vi "Main_MaintenanceCounters.vi"() -> ()   [LabVIEW 2017]
panel:
  in  "LastCycleTimeCluster":cluster{"MachineName":string, "LastHour":string}
  out "LastCycleTimePath":path
  in  "CycleTimeArray":T1(array[cluster])
  in  "LastSeconds":i32
  out "ThisAppPath":path
  out "ModificationArray":string[](array[string])
  out "HourResetEnabled":string
  out "CycleCountHour":T2
  in  "ArrayCycleCountHour":T3(array[cluster])
  out "UserLevel":i32
  out "ServerConnectionStatus":string
  out "Line Name":string
  out "Array_BooleanMemoryPLC":T4(array[cluster])
  out "UserLogged":string
  in  "FormatCountersConfigArray":T5(array[cluster]) {"StoppageAlarmCounter" format="%#_6f"; "PreparationAlarmCounter" format="%#_6f"}
  out "CycleTimeCluster":T6
  out "Table Control":string[][](table)
  out "ConnectionCluster":cluster{"Connection":bool, "MachineName":string}
  out "UDT_1":T7
  in  "CountersConfiguration":T8
  out "CountersConfigMerged":T5(array[cluster])
  out "CounterLineName Path":path
  in  "Tab":T9(tab)
  in  "RefreshLists":bool
  in  "Selector_P#-Description":u16(ring) items=["104567 - Spinning Belt", "108724 - Emergency Stop", "105855 - Helicoil", "101415 - Inductive Sensor", "101111 - Magnetic Sensor"]
  in  "Selector_MachineSpareParts":u16(ring) items=["MA530", "MA520", "MA500-3", "MA500-2", "MA500-1", "MA490-2", "MA490-1", "MA475", "MA470", "MA455", "MA336", "MA335", "SNX2030"]
  out "PathLocationMachineImage":path
  out "PathSparePartImage":path
  out "Image_LocationInMachine":T10(plugin-control)
  out "Image_SparePart":T10(plugin-control)
  in  "ModelName":u16(ring) items=["F042", "F070", "F0AU"]
  in  "Add Button":bool
  out "Description":string
  out "Tool Crib PN":string
  in  "SearchSpareParts":bool
  in  "CountersConfigArray":T5(array[cluster]) {"StoppageAlarmCounter" format="%#_6f"; "PreparationAlarmCounter" format="%#_6f"}
  in  "RefreshCountersConfig":bool
  in  "SaveCountersConfig":bool
  out "Counters Configuration Path":path
  in  "MachineNameID":u16(ring) items=["MA530", "MA520", "MA500-3", "MA500-2", "MA500-1", "MA490-2", "MA490-1", "MA475", "MA470", "MA455", "MA336", "MA335", "SNX2030"]
  in  "PLC Connection Array":T11(array[cluster]) {"PLC Type" items=["Keyence", "Allen Bradley", "Mitsubishi", "Panasonic", "Siemens"]}
  out "PLC Configuration Path":path
  in  "SavePLCConfig":bool
  in  "RefreshPLCConfig":bool
  in  "CreateTables":bool
  in  "EditUser":bool
  in  "GeneralParametersArray":cluster{"Parameter":string, "Value":string}[](array[cluster])
  in  "LoadDefaultConfig":bool
  in  "RemoveUser":bool
  in  "Logout":bool
  in  "Login":bool
  in  "AddUser":bool
  in  "GDrive":bool
  out "GeneralConfigPath":path
  in  "RefreshGeneralConfig":bool
  in  "SaveGeneralConfig":bool
  in  "ShowParetto":bool
  out "CycleTimeMonitor":T12(array[cluster])
  out "CycleTimePath":path
  out "legend":string[][](table)
  in  "Tab Control":T13(tab)
  in  "DictionaryArray":T14(array[cluster]) {"LifeCycle" format="%#_6f"}
  out "PathDictionary":path
  in  "SaveDictionary":bool
  in  "RefreshDictionary":bool
  in  "ResetAlarmButton":bool
  in  "QualityLogin":bool
  in  "MaintenanceLogin":bool
  in  "ResetAlarm":bool[](array[boolean])
  out "ArrayAlarm":bool[](array[boolean])
  out "OnlineStations":T15(array[cluster])
  in  "Counters Monitor Array":T16(array[cluster])
  out "CurrentCountersPath":path
  in  "Count Signal":bool[](array[boolean])
  in  "SaveCurrentCounter":bool
  in  "RefreshCurrentCounter":bool
  in  "Sort":bool
  out "Hour":string
  in  "stop":bool
  # "Cycles Based Maintenance"
  # "User"
  # "Line"
  # "Nidec Server Connection"
  # "Refresh Lists"
  # "Select Machine"
  # "Select PartNumber - Description"
  # "Location in the Machine"
  # "Spare Part Image"
  # "These paths are calculated automatically"
  # "Machine Name"
  # "Tool Crib P#"
  # "Description"
  # "SP1"
  # "SP2"
  # "Search Result"
  # "Model"
  # "Note:\nSP1 = Is the setpoint for the counter when the \nmachine will alert to prepare the replacement of\nthe component. This gives the technician time\nto get parts together.\n\nSP2 = Is the setpoint for the counter when the\nmachine will stop the operation until the part is \nreplaced, the operation can only be reset until\na quality employee comes to unlock with its \nuser and password."
  # "USER LEVEL 3 OR ABOVE TO ENABLE THIS CONFIGURATION IS NEEDED."
  # "Add the option to connect by serial port"
  # "Count Signal"
  # "Alarm Signal"
  # "Alarm Message"
  # "Machine Name"
  # "PLC Address"
  # "PLC Type"
  # "Value"
  # "Parameter"
  # "User Level 5 Requiered to View General Parameters"
  # "User Management"
  # "Idle Time: Is the maximum waiting time before a breakdown incidence is\nconsidered and created."
  # "Escalation Time: Is the maximum waiting time before sending an email \nto the escalation chain."
  # "Cycle Time Monitor"
  # "Cycle Time Monitor"
  # "Note: \nTo add a machine in this list of counters configuration it must be firt added in the PLC Connection tab."
  # "The SubAssembly can be either EOL, Motor, Stator, Rotor Etc, This is used to be able to crate several tables for the same line."
  # "buscar multiplos de ciclos para que coincidan \n\nestudiar investigacion de operaciones\n\nAgrupar las maquinas que trabajan en conjunto para agrupar tareas de mantenimiento.\nCambiar el metodo de seleccion de memorias de PLC usando solo strings para hacerlos universales."
  # "Nota para desarrollador: Revisar que al cerrar la incidencia se apague la alarma y se resetee el contador"
  # "1. Save counters to be loaded in the last state when the app starts up.\n\n2.Algorithm to read PLC counter values.\nthe key will be to set the signal from the PLC and reset from LabVIEW and the machine won't be able to start the new signal if the application has not been reset the previous one.\n\n3. Autosort getting the red status all the way up.\n\n4. Check cyle time between parts (The count signal must is the same for all the components in the same machine)"
  # "Component"
  # "Cycle Life"
  # "Manual"
  # "Un calculador de tiempo de vida en ciclos, que dependa del tipo de componente para calcular de acuerdo a la aplicacion.\n\npor ejemplo un slider, su tiempo de vida en es km de recorrido, midiendo cuanto se desplaza en cada movimiento, y cuantos desplazamientos hace por ciclo, se puede predecir, a los cuantos\nciclos va a fallar."
  # "Version:\nCBM V1.1\n03/03/2022 - 11:00\nEdgar Cruz\nMaintenance"
  # "Release Notes:\nV1.1 Will be able to support different PLC. since previous version only supports Keyence.\nFirts instance will be Allen Bradly to handle MK100."
  # "MachineName"
  # "Tool Crib"
  # "ComponentName"
  # "Counter SetPoint"
  # "Actual"
  # "Status"
  # "Online Stations"
  # "Current Hour"
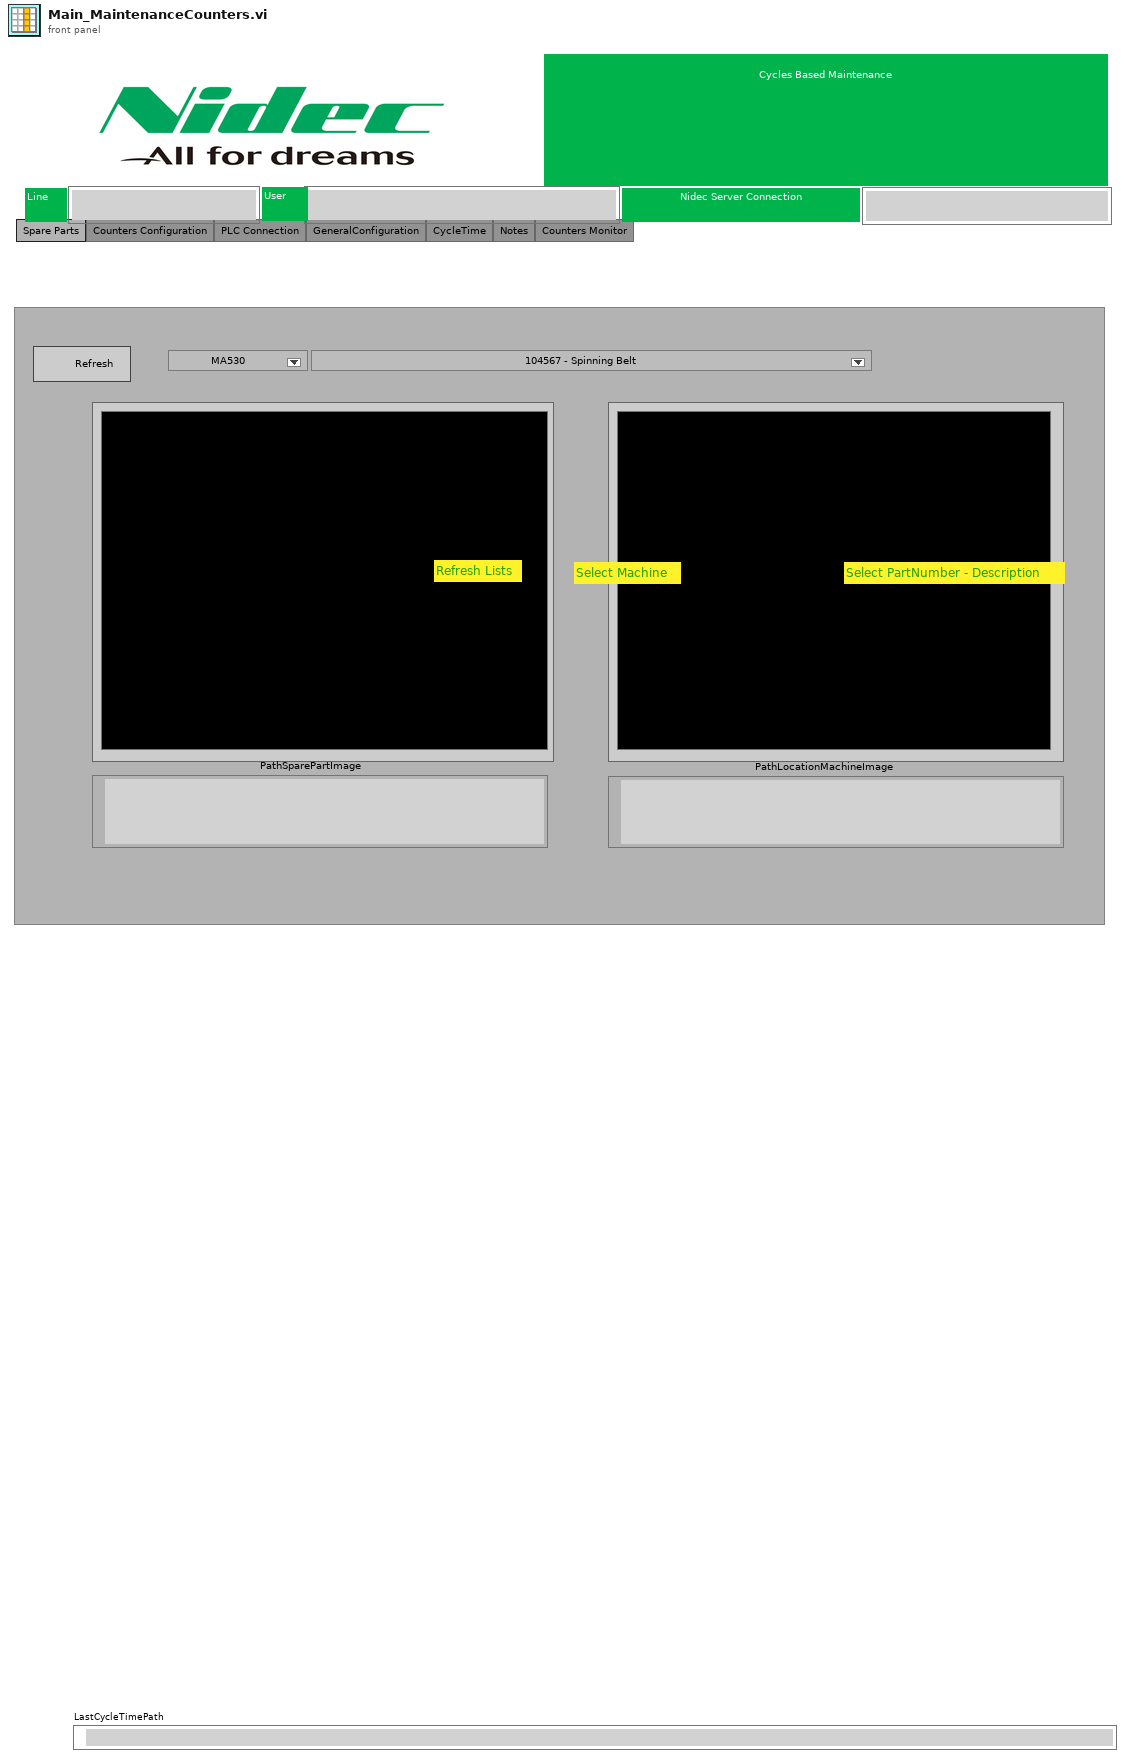
[diagram p1: front panel]
types:
  T1 = cluster{"MachineName":string, "LastHour":string}[]
  T2 = cluster{"MachineName":string, "HourLastCycle":string}
  T3 = cluster{"MachineName":string, "HourLastCycle":string}[]
  T4 = cluster{"PLC_Signal":bool, "MachineName":string}[]
  T5 = cluster{"ToolCribPartNumber":string, "ComponentName":string, "PreparationAlarmCounter":dbl, "StoppageAlarmCounter":dbl}[]
  T6 = cluster{"Connection":bool, "MachineName":string, "CycleTime":dbl}
  T7 = cluster{"ToolCribPartNumber":string, "ComponentName":string, "PreparationAlarmCounter":dbl, "StoppageAlarmCounter":dbl, "MachineName":string}
  T8 = cluster{"MachineName":string, "ComponentName":string, "StoppageAlarmCounter":dbl, "CurrentCount":dbl, "StatusColorBox":u32, "ToolCribPartNumber":string}
  T9 = enum32{"Spare Parts", "Counters Configuration", "PLC Connection", "GeneralConfiguration", "CycleTime", "Notes", "Counters Monitor"}
  T10 = typedef "IMAQ Image.ctl" = refnum<image>
  T11 = cluster{"MachineName":string, "PLC Address":string, "PLC Type":u16, "MemoryNumber1":string, "MemoryNumber2":string, "MemoryNumber3":string}[]
  T12 = cluster{"Connection":bool, "MachineName":string, "CycleTime":dbl}[]
  T13 = enum32{"Notes", "Dictionary", "Calculator", "Version Information"}
  T14 = cluster{"ComponentDescription":string, "LifeCycle":dbl, "ManualPDF":string}[]
  T15 = cluster{"Connection":bool, "MachineName":string}[]
  T16 = cluster{"MachineName":string, "ComponentName":string, "StoppageAlarmCounter":i32, "CurrentCount":i32, "StatusColorBox":u32, "ToolCribPartNumber":string}[]
  T17 = cluster{"ToolCribPartNumber":string, "ComponentName":string, "PreparationAlarmCounter":dbl, "StoppageAlarmCounter":dbl, "MachineName":string}[]
  T18 = cluster{"MachineName":string, "ComponentName":string, "StoppageAlarmCounter":i32, "CurrentCount":i32, "StatusColorBox":u32, "ToolCribPartNumber":string}
  T19 = enum8{"Enabled", "Disabled", "Disabled and Grayed Out"}
  T20 = typedef "Image Type" = u32
  T21 = cluster{"ToolCribPartNumber":string, "ComponentName":string, "PreparationAlarmCounter":dbl, "StoppageAlarmCounter":dbl}
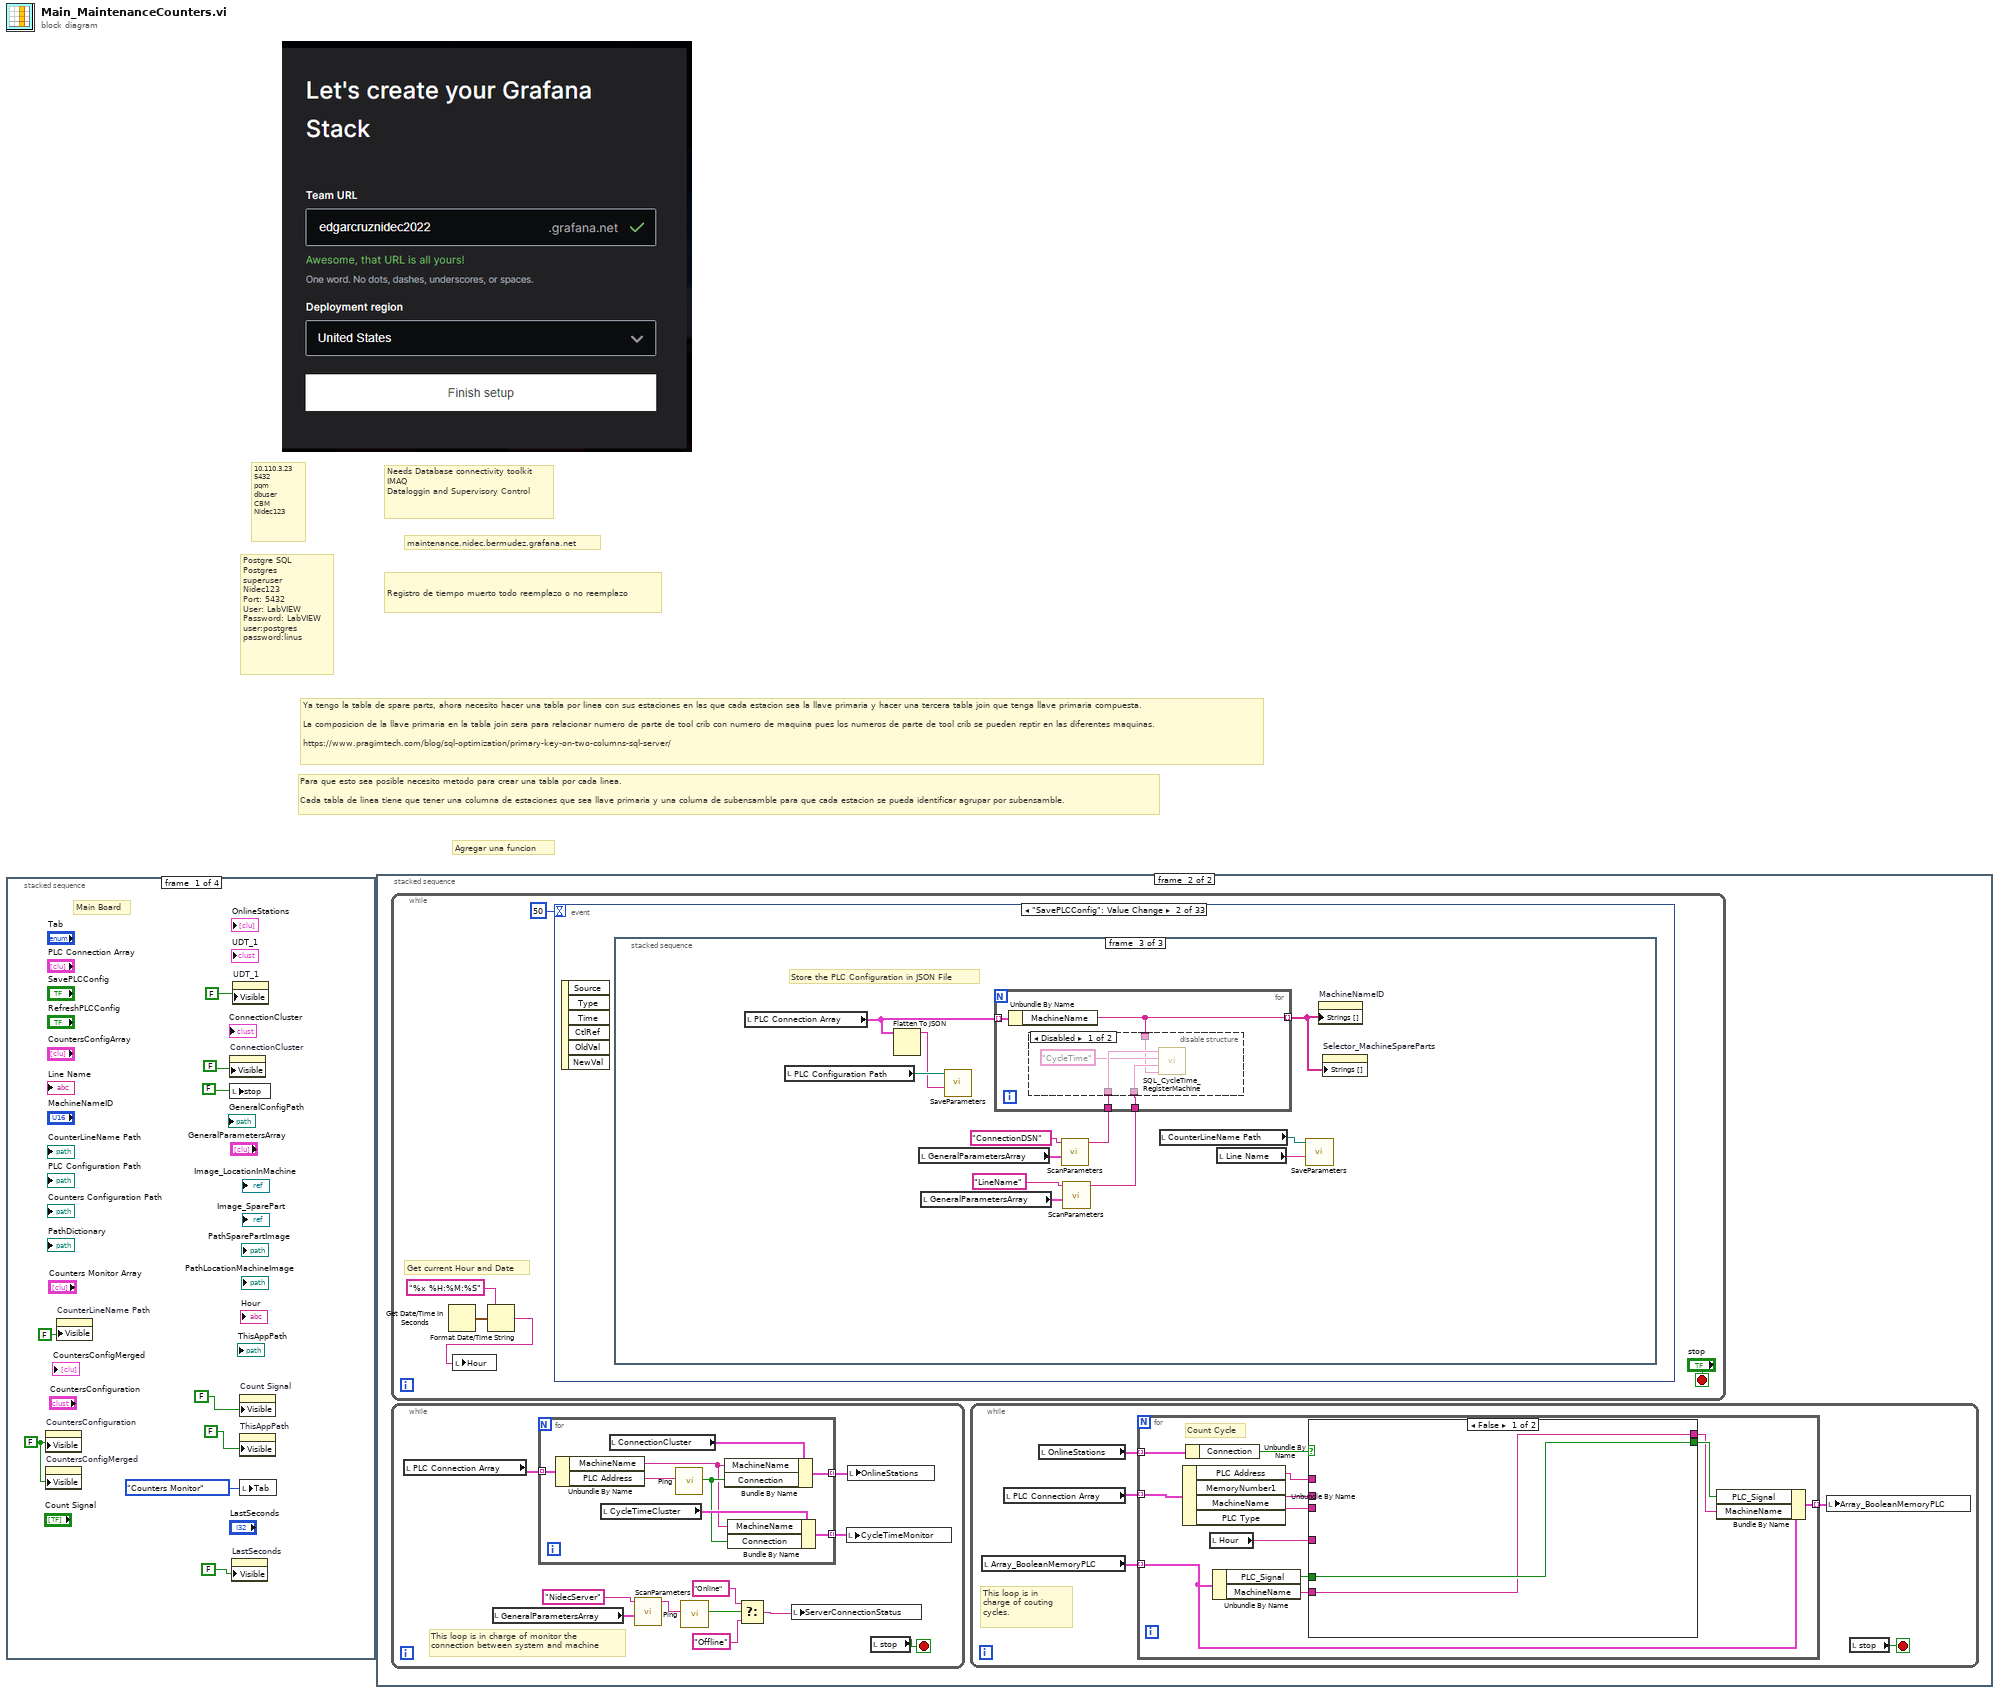
[diagram p0: block diagram]
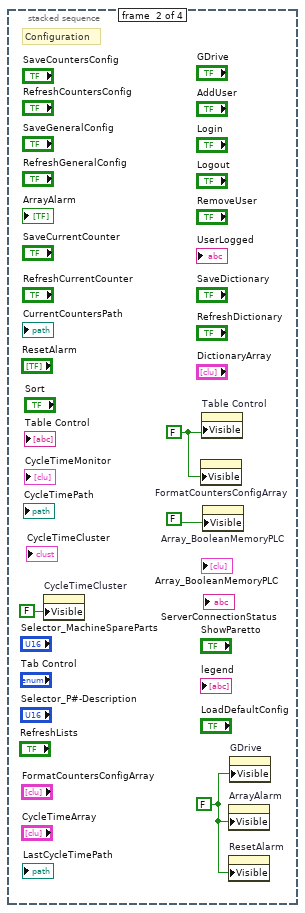
[diagram p2: hidden frame]
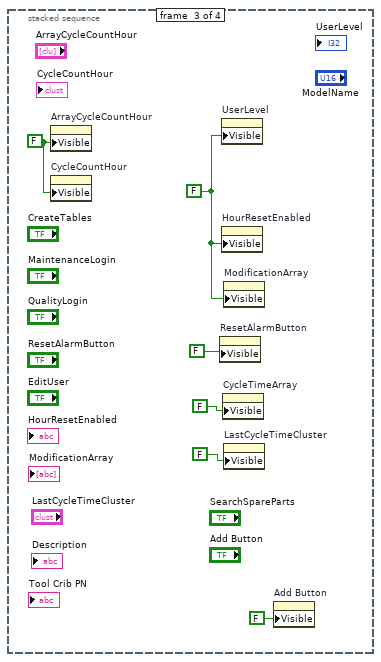
[diagram p3: hidden frame]
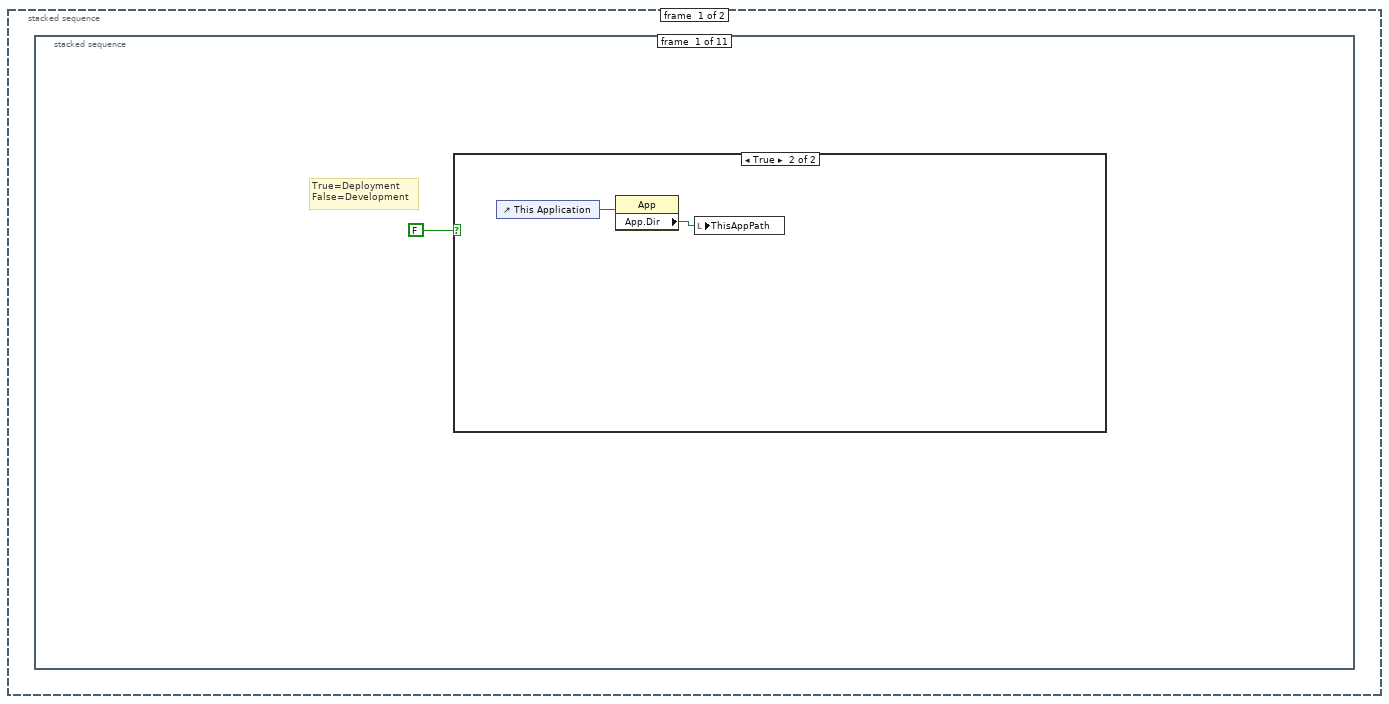
[diagram p5: hidden frame]
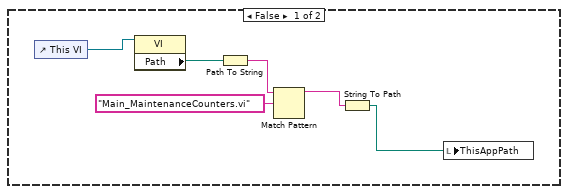
[diagram p6: hidden frame]
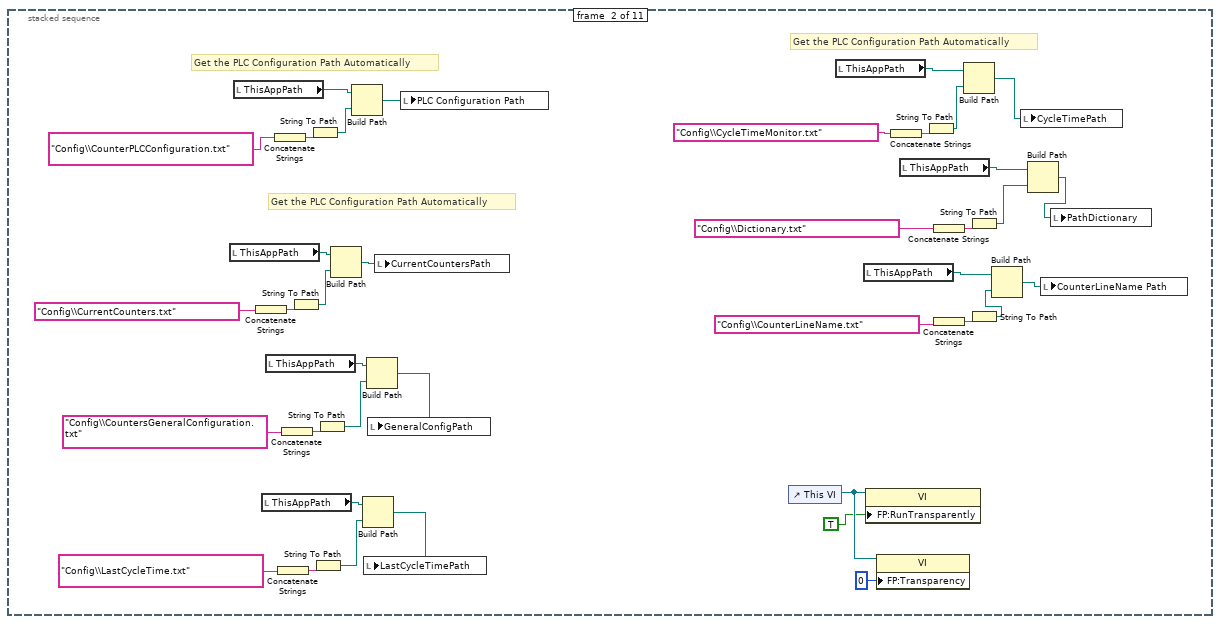
[diagram p7: hidden frame]
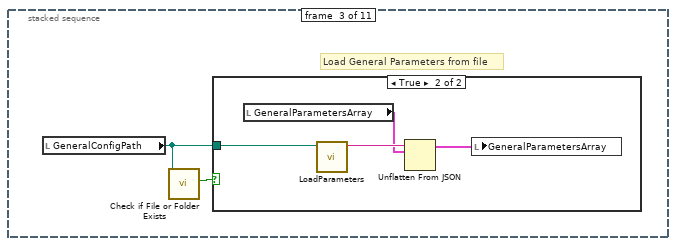
[diagram p8: hidden frame]
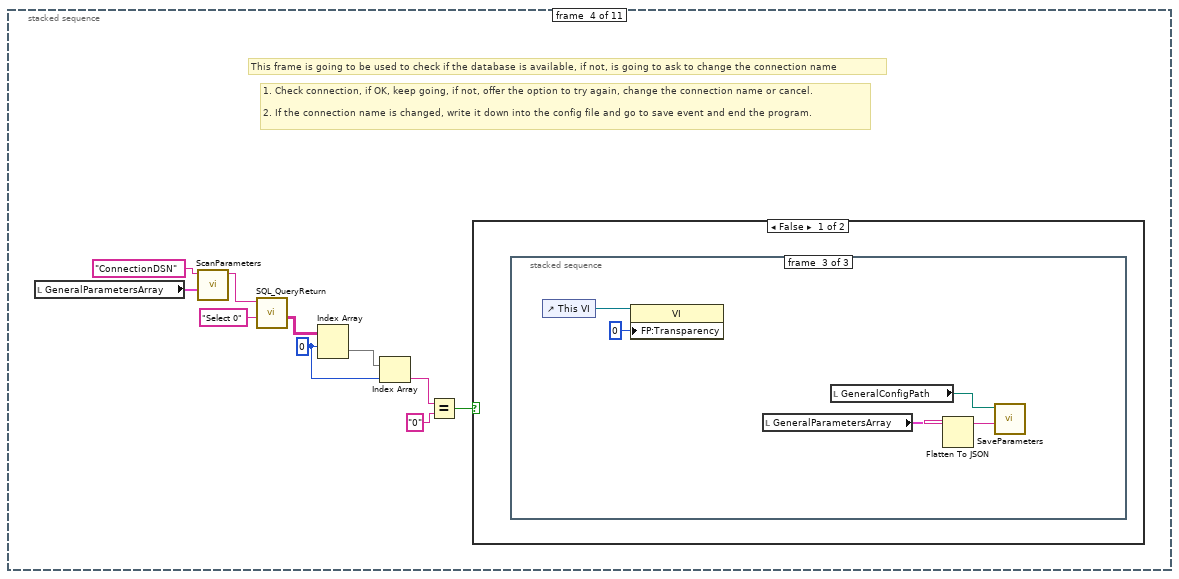
[diagram p10: hidden frame]
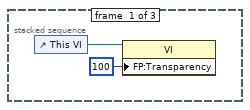
[diagram p11: hidden frame]
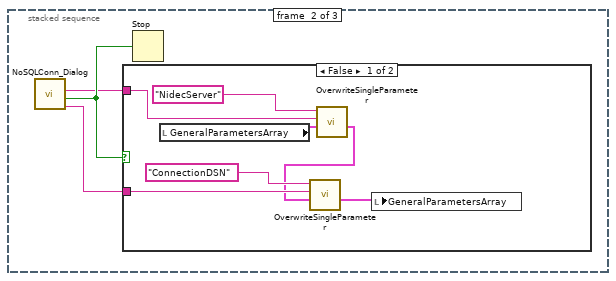
[diagram p12: hidden frame]
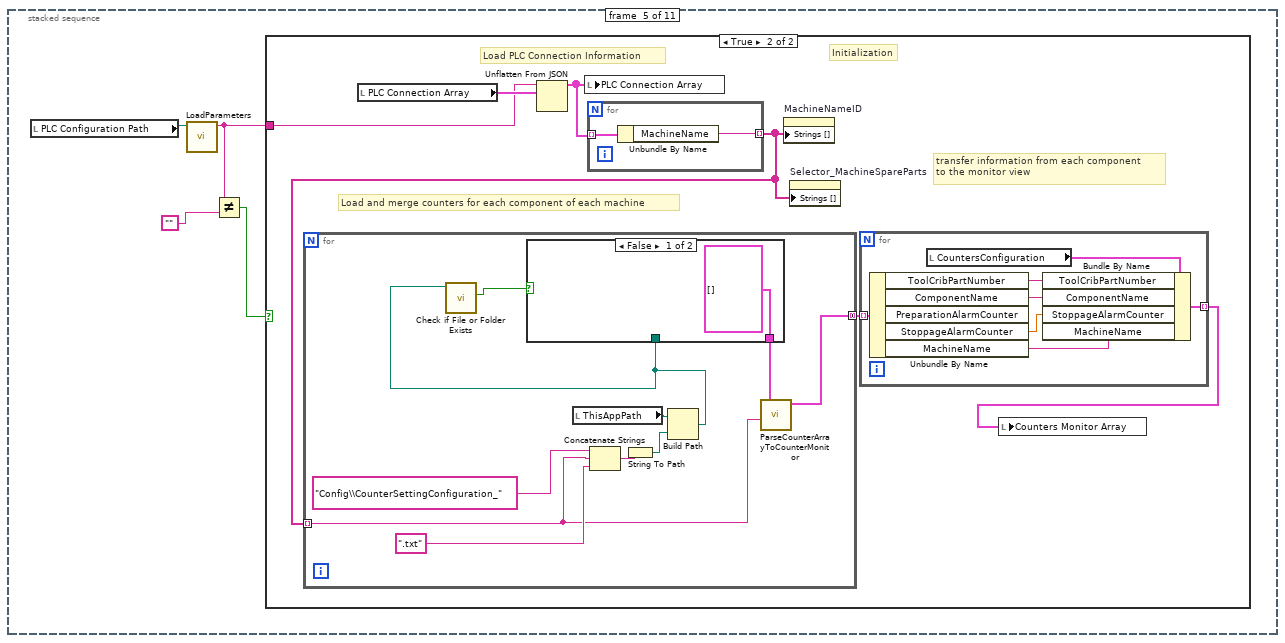
[diagram p15: hidden frame]
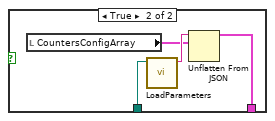
[diagram p17: hidden frame]
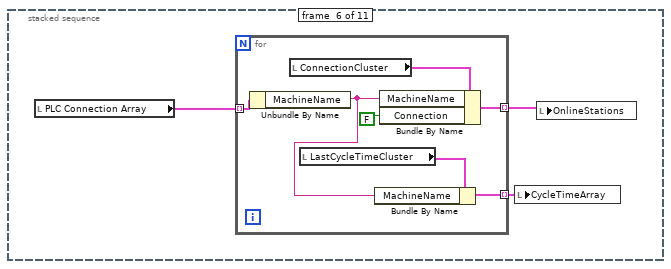
[diagram p18: hidden frame]
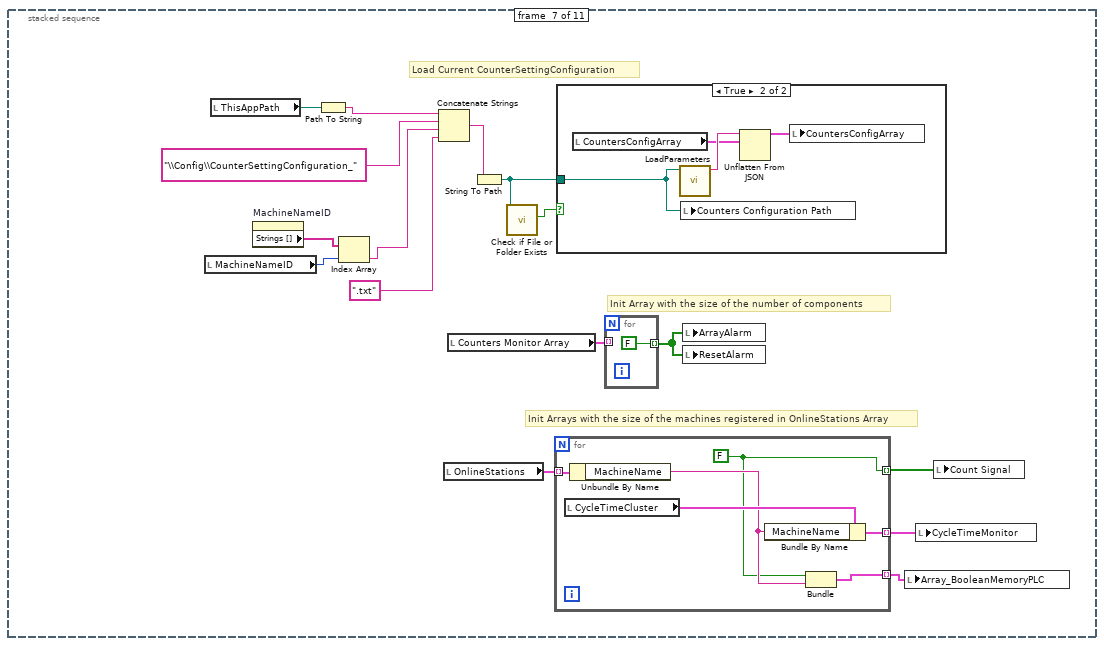
[diagram p19: hidden frame]
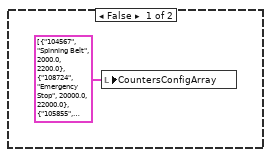
[diagram p20: hidden frame]
diagram:
  # "Agregar una funcion"
  # "Para que esto sea posible necesito metodo para crear una tabla por cada linea.\n\nCada tabla de linea tiene que tener una columna de estaciones que sea llave primaria y una columa de subensamble para que cada estacion se pueda identificar agrupar por subensamble."
  # "Ya tengo la tabla de spare parts, ahora necesito hacer una tabla por linea con sus estaciones en las que cada estacion sea la llave primaria y hacer una tercera tabla join que tenga llave primaria compuesta.\n\nLa composicion de la llave primaria en la tabla join sera para relacionar numero de parte de tool crib con numero de maquina pues los numeros de parte de tool crib se pueden reptir en las diferentes maquinas.\n\nhttps://www.pragimtech.com/blog/sql-optimization/primary-key-on-two-columns-sql-server/"
  # "10.110.3.23\n5432\npqm\ndbuser\nCBM\nNidec123"
  # "maintenance.nidec.bermudez.grafana.net"
  # "Needs Database connectivity toolkit\nIMAQ\nDataloggin and Supervisory Control"
  # "Registro de tiempo muerto todo reemplazo o no reemplazo"
  # "Postgre SQL \nPostgres\nsuperuser\nNidec123\nPort: 5432\nUser: LabVIEW\nPassword: LabVIEW\nuser:postgres\npassword:linus"
  n1 = stacked-sequence {
    frame #0 {
      w8 = FALSE
      # "Main Board"
      n2 = property on="CountersConfiguration" class="Clust (strict)"("Visible"=w8) -> ()  [unwired: 2 in, 2 out]
      n3 = property on="CountersConfigMerged" class="Arr (strict)"("Visible"=w8) -> ()  [unwired: 2 in, 2 out]
      n4 = property on="CounterLineName Path" class="Path"("Visible"=FALSE) -> ()  [unwired: 2 in, 2 out]
      n5 = property on="ConnectionCluster" class="Clust (strict)"("Visible"=FALSE) -> ()  [unwired: 2 in, 2 out]
      n6 = local write "stop"(FALSE ("stop")) -> ()
      n7 = property on="LastSeconds" class="DigNum (strict)"("Visible"=FALSE) -> ()  [unwired: 2 in, 2 out]
      n8 = property on="UDT_1" class="Clust (strict)"("Visible"=FALSE) -> ()  [unwired: 2 in, 2 out]
      n9 = property on="Count Signal" class="Arr (strict)"("Visible"=FALSE) -> ()  [unwired: 2 in, 2 out]
      n10 = property on="ThisAppPath" class="Path"("Visible"=FALSE) -> ()  [unwired: 2 in, 2 out]
      n11 = local write "Tab"(T9."Counters Monitor" ("Tab")) -> ()
    }
    frame #1 {
      w11 = FALSE ("Visible")
      w12 = FALSE ("Visible")
      # "Configuration"
      n12 = property on="CycleTimeCluster" class="Clust (strict)"("Visible"=FALSE) -> ()  [unwired: 2 in, 2 out]
      n13 = property on="FormatCountersConfigArray" class="Arr (strict)"("Visible"=w12) -> ()  [unwired: 2 in, 2 out]
      n14 = property on="Table Control" class="Tbl (strict)"("Visible"=w12) -> ()  [unwired: 2 in, 2 out]
      n15 = property on="Array_BooleanMemoryPLC" class="Arr (strict)"("Visible"=FALSE) -> ()  [unwired: 2 in, 2 out]
      n16 = property on="ArrayAlarm" class="Arr (strict)"("Visible"=w11) -> ()  [unwired: 2 in, 2 out]
      n17 = property on="ResetAlarm" class="Arr (strict)"("Visible"=w11) -> ()  [unwired: 2 in, 2 out]
      n18 = property on="GDrive" class="Bool"("Visible"=w11) -> ()  [unwired: 2 in, 2 out]
    }
    frame #2 {
      w19 = FALSE
      w18 = FALSE
      n19 = property on="ArrayCycleCountHour" class="Arr (strict)"("Visible"=w19) -> ()  [unwired: 2 in, 2 out]
      n20 = property on="CycleCountHour" class="Clust (strict)"("Visible"=w19) -> ()  [unwired: 2 in, 2 out]
      n21 = property on="ResetAlarmButton" class="Bool"("Visible"=FALSE) -> ()  [unwired: 2 in, 2 out]
      n22 = property on="UserLevel" class="DigNum (strict)"("Visible"=w18) -> ()  [unwired: 2 in, 2 out]
      n23 = property on="HourResetEnabled" class="Str"("Visible"=w18) -> ()  [unwired: 2 in, 2 out]
      n24 = property on="CycleTimeArray" class="Arr (strict)"("Visible"=FALSE) -> ()  [unwired: 2 in, 2 out]
      n25 = property on="ModificationArray" class="Arr (strict)"("Visible"=w18) -> ()  [unwired: 2 in, 2 out]
      n26 = property on="LastCycleTimeCluster" class="Clust (strict)"("Visible"=FALSE) -> ()  [unwired: 2 in, 2 out]
      n27 = property on="Add Button" class="Bool"("Visible"=FALSE) -> ()  [unwired: 2 in, 2 out]
    }
    frame #3 {
    }
  }
  n28 = stacked-sequence {
    frame #0 {
      n29 = stacked-sequence {
        frame #0 {
          # "True=Deployment\nFalse=Development"
          n30 = case shown="True" FALSE {
            frame False {
              n31 = control-ref of="This VI"() -> (w26:refnum<vi>)
              n32 = property class="VI"(reference=w26) -> ("Path"=w25:path)  [unwired: 1 in, 2 out]
              n33 = Path To String(path=w25) -> (string=w24:string)
              n34 = Match Pattern(string=w24, regular expression="Main_MaintenanceCounters.vi") -> (before substring=w22:string)  [unwired: 1 in, 3 out]
              n35 = String To Path(string=w22) -> (path=w21:path)
              n36 = local write "ThisAppPath"(w21) -> ()
            }
            frame True {
              n37 = control-ref of="This Application"() -> (w28:refnum<vi>)
              n38 = property class="App"(reference=w28) -> ("App.Dir"=w27:path)  [unwired: 1 in, 2 out]
              n39 = local write "ThisAppPath"(w27) -> ()
            }
          }
        }
        frame #1 {
          # "Get the PLC Configuration Path Automatically"
          # "Get the PLC Configuration Path Automatically"
          # "Get the PLC Configuration Path Automatically"
          n40 = local read "ThisAppPath"() -> (w48:path)
          n41 = local read "ThisAppPath"() -> (w50:path)
          n42 = Concatenate Strings("Config\\CurrentCounters.txt" ("regular expression")) -> (w63:string)
          n43 = local read "ThisAppPath"() -> (w31:path)
          n44 = local read "ThisAppPath"() -> (w45:path)
          n45 = Concatenate Strings("Config\\CounterPLCConfiguration.txt" ("regular expression")) -> (w66:string)
          n46 = Concatenate Strings("Config\\LastCycleTime.txt" ("regular expression")) -> (w29:string)
          n47 = Concatenate Strings("Config\\CountersGeneralConfiguration.txt" ("regular expression")) -> (w58:string)
          n48 = String To Path(string=w63) -> (path=w47:path)
          n49 = String To Path(string=w66) -> (path=w51:path)
          n50 = String To Path(string=w29) -> (path=w32:path)
          n51 = String To Path(string=w58) -> (path=w44:path)
          n52 = Build Path(base path=w48, name or relative path=w47) -> (appended path=w46:path)
          n53 = Build Path(base path=w50, name or relative path=w51) -> (appended path=w49:path)
          n54 = Build Path(base path=w31, name or relative path=w32) -> (appended path=w33:path)
          n55 = local write "LastCycleTimePath"(w33) -> ()
          n56 = Build Path(base path=w45, name or relative path=w44) -> (appended path=w43:path)
          n57 = local write "GeneralConfigPath"(w43) -> ()
          n58 = local write "CurrentCountersPath"(w46) -> ()
          n59 = local write "PLC Configuration Path"(w49) -> ()
          n60 = control-ref of="This VI"() -> (w54:refnum<vi>)
          n61 = local read "ThisAppPath"() -> (w42:path)
          n62 = local read "ThisAppPath"() -> (w36:path)
          n63 = property class="VI"(reference=w54, "FP:RunTransparently"=TRUE) -> ()  [unwired: 1 in, 2 out]
          n64 = property class="VI"(reference=w54, "FP:Transparency"=u8 0 ("Front Panel Window:Transparency")) -> ()  [unwired: 1 in, 2 out]
          n65 = Concatenate Strings("Config\\CycleTimeMonitor.txt" ("regular expression")) -> (w62:string)
          n66 = local read "ThisAppPath"() -> (w39:path)
          n67 = String To Path(string=w62) -> (path=w41:path)
          n68 = Concatenate Strings("Config\\Dictionary.txt" ("regular expression")) -> (w59:string)
          n69 = Concatenate Strings("Config\\CounterLineName.txt" ("regular expression")) -> (w56:string)
          n70 = Build Path(base path=w42, name or relative path=w41) -> (appended path=w40:path)
          n71 = String To Path(string=w59) -> (path=w38:path)
          n72 = String To Path(string=w56) -> (path=w35:path)
          n73 = Build Path(base path=w36, name or relative path=w35) -> (appended path=w34:path)
          n74 = local write "CycleTimePath"(w40) -> ()
          n75 = Build Path(base path=w39, name or relative path=w38) -> (appended path=w37:path)
          n76 = local write "CounterLineName Path"(w34) -> ()
          n77 = local write "PathDictionary"(w37) -> ()
        }
        frame #2 {
          # "Load General Parameters from file"
          n78 = local read "GeneralConfigPath"() -> (w67:path)
          n79 = call <vilib>:"Check if File or Folder Exists.vi"("path"=w67) -> ("file or folder exists?"=w68:bool)  [unwired: 8 in, 2 out]
          n80 = case shown="True" w68 {
            tunnel: w67 -> [_ w72]
            frame False {
            }
            frame True {
              n81 = local read "GeneralParametersArray"() -> (w70:cluster{"Parameter":string, "Value":string}[])
              n82 = call "LoadParameters.vi"("ShiftConfigPath"=w72) -> ("JSON_Text"=w71:string)  [unwired: 10 in]
              n83 = Unflatten From JSON(JSON string=w71, type and defaults=w70) -> (value=w69:cluster{"Parameter":string, "Value":string}[])  [unwired: 5 in, 1 out]
              n84 = local write "GeneralParametersArray"(w69) -> ()
            }
          }
        }
        frame #3 {
          w75 = 0 ("index (row)")
          # "1. Check connection, if OK, keep going, if not, offer the option to try again, change the connection name or cancel.\n\n2. If the connection name is changed, write it down into the config file and go to save event and end the program."
          # "This frame is going to be used to check if the database is available, if not, is going to ask to change the connection name"
          n85 = local read "GeneralParametersArray"() -> (w82:cluster{"Parameter":string, "Value":string}[])
          n86 = call "ScanParameters.vi"("MainConfigurationArray"=w82, "Parameter"="ConnectionDSN") -> ("Value"=w80:string)  [unwired: 9 in]
          n87 = call "SQL_QueryReturn.vi"("SQL query"="Select 0", "ConnectionDSN"=w80) -> ("data"=w78:string[][])  [unwired: 9 in]
          n88 = Index Array(array=w78, index (row)=w75) -> (element=w76:string[])  [unwired: 1 in]
          n89 = Index Array(array=w76, index=w75) -> (element=w74:string)
          n90 = Equal?(x=w74, y="0" ("SQL query")) -> (x = y?=w73:bool)
          n91 = case shown="False" w73 {
            frame False {
              n92 = stacked-sequence {
                frame #0 {
                  n93 = control-ref of="This VI"() -> (w83:refnum<vi>)
                  n94 = property class="VI"(reference=w83, "FP:Transparency"=u8 100 ("Front Panel Window:Transparency")) -> ()  [unwired: 1 in, 2 out]
                }
                frame #1 {
                  n95 = call "NoSQLConn_Dialog.vi"() -> ("NewDSN"=w87:string, "Boolean"=w86:bool, "NewIPAddress"=w85:string)  [unwired: 9 in]
                  n96 = case shown="False" w86 {
                    tunnel: w87 -> [w93 _]
                    tunnel: w85 -> [w90 _]
                    frame False {
                      n97 = local read "GeneralParametersArray"() -> (w91:cluster{"Parameter":string, "Value":string}[])
                      n98 = call "OverwriteSingleParameter.vi"("MainConfigurationArrayIN"=w91, "Value"=w90, "Parameter"="NidecServer") -> ("MainConfigurationArrayOUT"=w88:cluster{"Parameter":string, "Value":string}[])  [unwired: 8 in]
                      n99 = call "OverwriteSingleParameter.vi"("MainConfigurationArrayIN"=w88, "Value"=w93, "Parameter"="ConnectionDSN") -> ("MainConfigurationArrayOUT"=w89:cluster{"Parameter":string, "Value":string}[])  [unwired: 8 in]
                      n100 = local write "GeneralParametersArray"(w89) -> ()
                    }
                    frame True {
                    }
                  }
                  n101 = Stop(stop? (T)=w86) -> ()
                }
                frame #2 {
                  n102 = control-ref of="This VI"() -> (w99:refnum<vi>)
                  n103 = property class="VI"(reference=w99, "FP:Transparency"=u8 0 ("Front Panel Window:Transparency")) -> ()  [unwired: 1 in, 2 out]
                  n104 = local read "GeneralParametersArray"() -> (w95:cluster{"Parameter":string, "Value":string}[])
                  n105 = local read "GeneralConfigPath"() -> (w97:path)
                  n106 = Flatten To JSON(anything=w95) -> (JSON string=w96:string)  [unwired: 2 in, 1 out]
                  n107 = call "SaveParameters.vi"("JSON_Text"=w96, "ShiftConfigPath"=w97) -> ()  [unwired: 10 in]
                }
              }
            }
            frame True {
            }
          }
        }
        frame #4 {
          n108 = local read "PLC Configuration Path"() -> (w103:path)
          n109 = call "LoadParameters.vi"("ShiftConfigPath"=w103) -> ("JSON_Text"=w102:string)  [unwired: 10 in]
          n110 = Not Equal?(x=w102, y="") -> (x != y?=w100:bool)
          n111 = case shown="True" w100 {
            tunnel: w102 -> [_ w104]
            frame False {
            }
            frame True {
              # "Initialization"
              # "transfer information from each component\nto the monitor view"
              # "Load and merge counters for each component of each machine"
              # "Load PLC Connection Information"
              n112 = local read "PLC Connection Array"() -> (w109:T11)
              n113 = Unflatten From JSON(JSON string=w104, type and defaults=w109) -> (value=w108:T11)  [unwired: 5 in, 1 out]
              n114 = local write "PLC Connection Array"(w108) -> ()
              n115 = for {
                tunnel: w108 -> [w132] mode=indexing
                tunnel: [w133] -> w105 mode=indexing
                n116 = Unbundle By Name(w132) -> ("MachineName"=w133:string)
              }
              n117 = for {
                tunnel: w105 -> [w123] mode=indexing
                tunnel: [w122] -> w106 mode=concatenating
                n118 = local read "ThisAppPath"() -> (w119:path)
                n119 = Concatenate Strings("Config\\CounterSettingConfiguration_" ("regular expression"), w123, ".txt" ("regular expression")) -> (w126:string)
                n120 = String To Path(string=w126) -> (path=w118:path)
                n121 = Build Path(base path=w119, name or relative path=w118) -> (appended path=w117:path)
                n122 = call <vilib>:"Check if File or Folder Exists.vi"("path"=w117) -> ("file or folder exists?"=w121:bool)  [unwired: 8 in, 2 out]
                n123 = case shown="False" w121 {
                  tunnel: [T5 [] ("CountersConfigArray") w130] -> w120
                  tunnel: w117 -> [_ w129]
                  frame False {
                  }
                  frame True {
                    n124 = local read "CountersConfigArray"() -> (w128:T5)
                    n125 = call "LoadParameters.vi"("ShiftConfigPath"=w129) -> ("JSON_Text"=w131:string)  [unwired: 10 in]
                    n126 = Unflatten From JSON(JSON string=w131, type and defaults=w128) -> (value=w130:T5)  [unwired: 5 in, 1 out]
                  }
                }
                n127 = call "ParseCounterArrayToCounterMonitor.vi"("MachineID"=w123, "CountersConfigArray"=w120) -> ("CounterMonitorArray"=w122:T17)  [unwired: 9 in]
              }
              n128 = property on="MachineNameID" class="Ring (strict)"("Strings []"=w105) -> ()  [unwired: 2 in, 2 out]
              n129 = property on="Selector_MachineSpareParts" class="Ring (strict)"("Strings []"=w105) -> ()  [unwired: 2 in, 2 out]
              n130 = for {
                tunnel: [w114] -> w107 mode=indexing
                tunnel: w106 -> [w113] mode=indexing
                n131 = Unbundle By Name(w113) -> ("ToolCribPartNumber"=w112:string, "ComponentName"=w115:string, "StoppageAlarmCounter"=w111:dbl, "MachineName"=w110:string)  [unwired: 1 out]
                n132 = local read "CountersConfiguration"() -> (w116:T8)
                n133 = Bundle By Name(cluster=w116, "ToolCribPartNumber"=w112, "ComponentName"=w115, "StoppageAlarmCounter"=w111, "MachineName"=w110) -> (w114:T8)
              }
              n134 = local write "Counters Monitor Array"(w107) -> ()
            }
          }
        }
        frame #5 {
          n135 = local read "PLC Connection Array"() -> (w136:T11)
          n136 = for {
            tunnel: w136 -> [w143] mode=indexing
            tunnel: [w141] -> w135 mode=indexing
            tunnel: [w137] -> w134 mode=indexing
            n137 = Unbundle By Name(w143) -> ("MachineName"=w138:string)
            n138 = local read "ConnectionCluster"() -> (w142:cluster{"Connection":bool, "MachineName":string})
            n139 = local read "LastCycleTimeCluster"() -> (w139:cluster{"MachineName":string, "LastHour":string})
            n140 = Bundle By Name(cluster=w139, "MachineName"=w138) -> (w137:cluster{"MachineName":string, "LastHour":string})
            n141 = Bundle By Name(cluster=w142, "MachineName"=w138, "Connection"=FALSE) -> (w141:cluster{"Connection":bool, "MachineName":string})
          }
          n142 = local write "CycleTimeArray"(w134) -> ()
          n143 = local write "OnlineStations"(w135) -> ()
        }
        frame #6 {
          # "Load Current CounterSettingConfiguration"
          # "Init Array with the size of the number of components"
          # "Init Arrays with the size of the machines registered in OnlineStations Array"
          n144 = local read "MachineNameID"() -> (w159:u16)
          n145 = local read "ThisAppPath"() -> (w144:path)
          n146 = property on="MachineNameID" class="Ring (strict)"() -> ("Strings []"=w158:string[])  [unwired: 2 in, 2 out]
          n147 = Path To String(path=w144) -> (string=w145:string)
          n148 = Index Array(array=w158, index=w159) -> (element=w156:string)
          n149 = Concatenate Strings(w145, "\\Config\\CounterSettingConfiguration_" ("regular expression"), w156, ".txt" ("regular expression")) -> (w157:string)
          n150 = local read "OnlineStations"() -> (w149:T15)
          n151 = local read "Counters Monitor Array"() -> (w151:T16)
          n152 = String To Path(string=w157) -> (path=w154:path)
          n153 = call <vilib>:"Check if File or Folder Exists.vi"("path"=w154) -> ("file or folder exists?"=w155:bool)  [unwired: 8 in, 2 out]
          n154 = for {
            tunnel: w149 -> [w164] mode=indexing
            tunnel: [w161] -> w148 mode=indexing
            tunnel: [w163] -> w147 mode=indexing
            tunnel: [w160] -> w146 mode=indexing
            w161 = FALSE
            n155 = local read "CycleTimeCluster"() -> (w165:T6)
            n156 = Unbundle By Name(w164) -> ("MachineName"=w162:string)
            n157 = Bundle By Name(cluster=w165, "MachineName"=w162) -> (w163:T6)
            n158 = Bundle(w161, "MachineName"=w162) -> (w160:cluster{bool, "MachineName":string})  [unwired: 1 in]
          }
          n159 = case shown="True" w155 {
            tunnel: w154 -> [_ w170]
            frame False {
              n160 = local write "CountersConfigArray"(T5 [{"ToolCribPartNumber"="104567", "ComponentName"="Spinning Belt", "PreparationAlarmCounter"=2000.0, "StoppageAlarmCounter"=2200.0}, {"ToolCribPartNumber"="108724", "ComponentName"="Emergency Stop", "PreparationAlarmCounter"=20000.0, "StoppageAlarmCounter"=22000.0}, {"ToolCribPartNumber"="105855", "ComponentName"="Helicoil", "PreparationAlarmCounter"=38000.0, "StoppageAlarmCounter"=40000.0}, {"ToolCribPartNumber"="101415", "ComponentName"="NewPart", "PreparationAlarmCounter"=12000.0, "StoppageAlarmCounter"=12300.0}] ("CountersConfigArray")) -> ()
            }
            frame True {
              n161 = local read "CountersConfigArray"() -> (w169:T5)
              n162 = call "LoadParameters.vi"("ShiftConfigPath"=w170) -> ("JSON_Text"=w171:string)  [unwired: 10 in]
              n163 = local write "Counters Configuration Path"(w170) -> ()
              n164 = Unflatten From JSON(JSON string=w171, type and defaults=w169) -> (value=w168:T5)  [unwired: 5 in, 1 out]
              n165 = local write "CountersConfigArray"(w168) -> ()
            }
          }
          n166 = for {
            tunnel: w151 -> [_] mode=indexing
            tunnel: [FALSE] -> w150 mode=indexing
          }
          n167 = local write "ArrayAlarm"(w150) -> ()
          n168 = local write "ResetAlarm"(w150) -> ()
          n169 = local write "Array_BooleanMemoryPLC"(w146) -> ()
          n170 = local write "CycleTimeMonitor"(w147) -> ()
          n171 = local write "Count Signal"(w148) -> ()
        }
        frame #7 {
          # "Load Dictionary"
          n172 = local read "CurrentCountersPath"() -> (w178:path)
          n173 = local read "Counters Monitor Array"() -> (w176:T16)
          n174 = local read "PathDictionary"() -> (w172:path)
          n175 = call "LoadParameters.vi"("ShiftConfigPath"=w178) -> ("JSON_Text"=w177:string)  [unwired: 10 in]
          n176 = call <vilib>:"Check if File or Folder Exists.vi"("path"=w172) -> ("file or folder exists?"=w173:bool)  [unwired: 8 in, 2 out]
          n177 = Unflatten From JSON(JSON string=w177, type and defaults=w176) -> (value=w175:T16)  [unwired: 5 in, 1 out]
          n178 = for {
            tunnel: w176 -> [w184] mode=indexing
            tunnel: w175 -> [w185]
            tunnel: [w183] -> w174 mode=indexing
            n179 = Unbundle By Name(w184) -> ("MachineName"=w188:string, "ComponentName"=w187:string, "ToolCribPartNumber"=w186:string)
            n180 = for {
              tunnel: w188 -> [w201]
              tunnel: w187 -> [w200]
              tunnel: w186 -> [w199]
              tunnel: w185 -> [w202] mode=indexing
              shift-right: [w189] -> w183
              shift-left: w184 -> [w190]
              n181 = Unbundle By Name(w202) -> ("MachineName"=w191:string, "ComponentName"=w192:string, "ToolCribPartNumber"=w193:string, "CurrentCount"=w195:i32)
              n182 = Equal?(x=w201, y=w191) -> (x = y?=w197:bool)
              n183 = Equal?(x=w200, y=w192) -> (x = y?=w198:bool)
              n184 = Equal?(x=w199, y=w193) -> (x = y?=w196:bool)
              n185 = Compound Arithmetic op=AND(w197, w198, w196) -> (w194:bool)
              n186 = case shown="True" w194 {
                tunnel: w195 -> [_ w209]
                tunnel: w193 -> [_ w208]
                tunnel: w192 -> [_ w207]
                tunnel: w191 -> [_ w206]
                tunnel: w190 -> [w203 w205]
                tunnel: [w203 w204] -> w189
                frame False {
                }
                frame True {
                  n187 = Bundle By Name(cluster=w205, "MachineName"=w206, "ComponentName"=w207, "ToolCribPartNumber"=w208, "CurrentCount"=w209) -> (w204:T18)
                }
              }
            }
          }
          n188 = case shown="True" w173 {
            tunnel: w172 -> [_ w181]
            frame False {
            }
            frame True {
              n189 = local read "DictionaryArray"() -> (w182:T14)
              n190 = call "LoadParameters.vi"("ShiftConfigPath"=w181) -> ("JSON_Text"=w180:string)  [unwired: 10 in]
              n191 = Unflatten From JSON(JSON string=w180, type and defaults=w182) -> (value=w179:T14)  [unwired: 5 in, 1 out]
              n192 = local write "DictionaryArray"(w179) -> ()
            }
          }
          n193 = local write "Counters Monitor Array"(w174) -> ()
        }
        frame #8 {
          w214 = T19."Disabled and Grayed Out" ("Disabled")
          # "Logout and disable information"
          # "Load Line name from General parameters"
          n194 = local write "UserLevel"(0) -> ()
          n195 = local write "UserLogged"("") -> ()
          n196 = property on="PLC Connection Array" class="Arr (strict)"("DisabledEnum"=w214) -> ()  [unwired: 2 in, 2 out]
          n197 = property on="GeneralParametersArray" class="Arr (strict)"("Visible"=FALSE) -> ()  [unwired: 2 in, 2 out]
          n198 = property on="CountersConfigArray" class="Arr (strict)"("DisabledEnum"=w214) -> ()  [unwired: 2 in, 2 out]
          n199 = local read "GeneralParametersArray"() -> (w211:cluster{"Parameter":string, "Value":string}[])
          n200 = call "ScanParameters.vi"("MainConfigurationArray"=w211, "Parameter"="LineName") -> ("Value"=w212:string)  [unwired: 9 in]
          n201 = local write "Line Name"(w212) -> ()
        }
        frame #9 {
          # "This array must have one element per machine and register the hour \nso it must be initialized with the number of stations"
          n202 = local read "OnlineStations"() -> (w232:T15)
          n203 = for {
            tunnel: w232 -> [w236] mode=indexing
            tunnel: [w233] -> w231 mode=indexing
            n204 = Unbundle By Name(w236) -> ("MachineName"=w234:string)
            n205 = local read "CycleCountHour"() -> (w235:T2)
            n206 = Bundle By Name(cluster=w235, "MachineName"=w234) -> (w233:T2)
          }
          n207 = local read "GeneralParametersArray"() -> (w224:cluster{"Parameter":string, "Value":string}[])
          n208 = local read "GeneralParametersArray"() -> (w223:cluster{"Parameter":string, "Value":string}[])
          n209 = local write "ArrayCycleCountHour"(w231) -> ()
          n210 = local read "GeneralParametersArray"() -> (w229:cluster{"Parameter":string, "Value":string}[])
          n211 = call "ScanParameters.vi"("MainConfigurationArray"=w224, "Parameter"="LineName") -> ("Value"=w225:string)  [unwired: 9 in]
          n212 = call "ScanParameters.vi"("MainConfigurationArray"=w223, "Parameter"="SubAssembly") -> ("Value"=w226:string)  [unwired: 9 in]
          n213 = Concatenate Strings("update \"", w225, "_userlogged\" set \"useroperations\"='0',\"userquality\"='0' where \"subassembly\"='", w226, "'") -> (w227:string)
          n214 = call "ScanParameters.vi"("MainConfigurationArray"=w229, "Parameter"="ConnectionDSN") -> ("Value"=w230:string)  [unwired: 9 in]
          n215 = To Lower Case(string=w227) -> (all lower case string=w228:string)
          n216 = call "SQL_QueryNoReturn.vi"("SQL query"=w228, "ConnectionDSN"=w230) -> ()  [unwired: 10 in]
        }
        frame #10 {
          n217 = local read "GeneralParametersArray"() -> (w240:cluster{"Parameter":string, "Value":string}[])
          n218 = local read "GeneralParametersArray"() -> (w242:cluster{"Parameter":string, "Value":string}[])
          n219 = local read "GeneralParametersArray"() -> (w246:cluster{"Parameter":string, "Value":string}[])
          n220 = local read "Counters Monitor Array"() -> (w237:T16)
          n221 = call "ScanParameters.vi"("MainConfigurationArray"=w240, "Parameter"="SubAssembly") -> ("Value"=w238:string)  [unwired: 9 in]
          n222 = call "ScanParameters.vi"("MainConfigurationArray"=w242, "Parameter"="LineName") -> ("Value"=w241:string)  [unwired: 9 in]
          n223 = call "ScanParameters.vi"("MainConfigurationArray"=w246, "Parameter"="ConnectionDSN") -> ("Value"=w244:string)  [unwired: 9 in]
          n224 = call "SQL_StoreCountersMonitor.vi"("Counters Monitor Array"=w237, "SubAssembly"=w238, "LineName"=w241, "ConnectionDSN"=w244) -> ()  [unwired: 8 in]
        }
      }
    }
    frame #1 {
      n225 = while {
        stop <- "stop" stop-if-true
        # "Get current Hour and Date"
        n226 = Get Date/Time In Seconds() -> (seconds since 1Jan1904=w308:timestamp)
        n227 = Format Date/Time String(time format string (%c)="%x %H:%M:%S", seconds (now)=w308) -> (date/time string=w305:string)  [unwired: 1 in]
        n228 = local write "Hour"(w305) -> ()
        n229 = event shown="[1] \"SavePLCConfig\": Value Change" {
          selector: _ -> [_ _ _ _ _ _ _ _ _ _ _ _ _ _ _ _ _ _ _ _ _ _ _ _ _ _ _ _ _ _ _ _ _]
          dyn-events: _ -> [_ _ _ _ _ _ _ _ _ _ _ _ _ _ _ _ _ _ _ _ _ _ _ _ _ _ _ _ _ _ _ _ _]
          timeout: 50 -> [_ _ _ _ _ _ _ _ _ _ _ _ _ _ _ _ _ _ _ _ _ _ _ _ _ _ _ _ _ _ _ _ _]
          event Timeout {
            n230 = event-data() -> ()  [unwired: 1 in, 3 out]
            n231 = stacked-sequence {
              frame #0 {
                # "Continuously store the Current Counters Montior in a File"
                # "Change the status indicator in the Counters Monitor and Send an Email in case any indicator is Red"
                n232 = local read "Counters Monitor Array"() -> (w331:T16)
                n233 = local read "GeneralParametersArray"() -> (w322:cluster{"Parameter":string, "Value":string}[])
                n234 = local read "GeneralParametersArray"() -> (w313:cluster{"Parameter":string, "Value":string}[])
                n235 = local read "GeneralParametersArray"() -> (w321:cluster{"Parameter":string, "Value":string}[])
                n236 = local read "GeneralParametersArray"() -> (w318:cluster{"Parameter":string, "Value":string}[])
                n237 = local read "GeneralParametersArray"() -> (w326:cluster{"Parameter":string, "Value":string}[])
                n238 = local read "ArrayAlarm"() -> (w328:bool[])
                n239 = call "ScanParameters.vi"("MainConfigurationArray"=w322, "Parameter"="SenderMail") -> ("Value"=w317:string)  [unwired: 9 in]
                n240 = call "ScanParameters.vi"("MainConfigurationArray"=w313, "Parameter"="ConnectionDSN") -> ("Value"=w311:string)  [unwired: 9 in]
                n241 = call "ScanParameters.vi"("MainConfigurationArray"=w321, "Parameter"="Password") -> ("Value"=w316:string)  [unwired: 9 in]
                n242 = call "ScanParameters.vi"("MainConfigurationArray"=w318, "Parameter"="Recipients") -> ("Value"=w315:string)  [unwired: 9 in]
                n243 = call "ScanParameters.vi"("MainConfigurationArray"=w326, "Parameter"="EmailsEnabled") -> ("Value"=w324:string)  [unwired: 9 in]
                n244 = local read "PLC Connection Array"() -> (w310:T11)
                n245 = local read "Line Name"() -> (w329:string)
                n246 = local read "OnlineStations"() -> (w314:T15)
                n247 = call "CountersVisualization.vi"("Counters Monitor Array IN"=w331, "SenderMail"=w317, "ConnectionDSN"=w311, "Password"=w316, "Recipients"=w315, "ArrayAlarmIN"=w328, "LineName"=w329, "PLC Connection Array"=w310, "OnlineStations"=w314, "EmailsEnabled"=w324) -> ("Counters Monitor Array OUT"=w330:T16, "ArrayAlarmOUT"=w327:bool[])  [unwired: 8 in]
                n248 = local write "Counters Monitor Array"(w330) -> ()
                n249 = local write "ArrayAlarm"(w327) -> ()
                n250 = local read "Counters Monitor Array"() -> (w332:T16)
                n251 = local read "CurrentCountersPath"() -> (w334:path)
                n252 = Flatten To JSON(anything=w332) -> (JSON string=w333:string)  [unwired: 2 in, 1 out]
                n253 = call "SaveParameters.vi"("JSON_Text"=w333, "ShiftConfigPath"=w334) -> ()  [unwired: 10 in]
              }
              frame #1 {
                # "If the usser logged in is level 5, enables all the configurations"
                n254 = local read "UserLevel"() -> (w338:i32)
                n255 = Greater Or Equal?(x=w338, y=3) -> (x >= y?=w335:bool)
                n256 = case shown="True" w335 {
                  frame False {
                  }
                  frame True {
                    w339 = T19."Enabled" ("Disabled")
                    n257 = property on="PLC Connection Array" class="Arr (strict)"("DisabledEnum"=w339) -> ()  [unwired: 2 in, 2 out]
                    n258 = property on="CountersConfigArray" class="Arr (strict)"("DisabledEnum"=w339) -> ()  [unwired: 2 in, 2 out]
                  }
                }
                n259 = property on="GeneralParametersArray" class="Arr (strict)"("Visible"=w335) -> ()  [unwired: 2 in, 2 out]
                n260 = property on="CreateTables" class="Bool"("Visible"=w335) -> ()  [unwired: 2 in, 2 out]
                n261 = property on="EditUser" class="Bool"("Visible"=w335) -> ()  [unwired: 2 in, 2 out]
                n262 = property on="LoadDefaultConfig" class="Bool"("Visible"=w335) -> ()  [unwired: 2 in, 2 out]
                n263 = property on="Add Button" class="Bool"("Visible"=w335) -> ()  [unwired: 2 in, 2 out]
                n264 = property on="ResetAlarmButton" class="Bool"() -> ("Visible"=w336:bool)  [unwired: 2 in, 2 out]
                n265 = case shown="True" w336 {
                  frame False {
                  }
                  frame True {
                    n266 = stacked-sequence {
                      seq-local: [w348 _ _] -> [_ w364 _]
                      seq-local: [w344 _ _] -> [_ w363 _]
                      seq-local: [w341 _ _] -> [_ w362 _]
                      seq-local: [w347 _ _] -> [_ w361 _]
                      frame #0 {
                        n267 = local read "HourResetEnabled"() -> (w352:string)
                        n268 = local read "Hour"() -> (w360:string)
                        n269 = call <vilib>:"Space Constant.vi"() -> ("String"=w359:string)
                        n270 = call <vilib>:"Space Constant.vi"() -> ("String"=w353:string)
                        n271 = Match Pattern(string=w360, regular expression=w359) -> (after substring=w358:string)  [unwired: 1 in, 3 out]
                        n272 = Match Pattern(string=w352, regular expression=w353) -> (after substring=w354:string)  [unwired: 1 in, 3 out]
                        n273 = Match Pattern(string=w358, regular expression=":" ("time format string (%c)")) -> (before substring=w356:string, after substring=w346:string)  [unwired: 1 in, 2 out]
                        n274 = Match Pattern(string=w354, regular expression=":" ("time format string (%c)")) -> (before substring=w342:string, after substring=w340:string)  [unwired: 1 in, 2 out]
                        n275 = Match Pattern(string=w346, regular expression=":" ("time format string (%c)")) -> (before substring=w344:string)  [unwired: 1 in, 3 out]
                        n276 = Decimal String To Number(string=w356) -> (number=w351:i32)  [unwired: 2 in, 1 out]
                        n277 = Decimal String To Number(string=w342) -> (number=w350:i32)  [unwired: 2 in, 1 out]
                        n278 = Match Pattern(string=w340, regular expression=":" ("time format string (%c)")) -> (before substring=w341:string)  [unwired: 1 in, 3 out]
                        n279 = Subtract(x=w351, y=w350) -> (x-y=w347:i32)
                        n280 = Equal?(x=w347, y=0) -> (x = y?=w348:bool)
                      }
                      frame #1 {
                        # "Difference in hours"
                        # "Enabled minute"
                        # "Current minute"
                        n281 = case shown="True" w364 {
                          tunnel: w363 -> [w373 w391]
                          tunnel: w362 -> [w374 w390]
                          tunnel: w361 -> [w380 _]
                          frame False {
                            n282 = Match Pattern(string=w374, regular expression=":" ("time format string (%c)")) -> (before substring=w377:string)  [unwired: 1 in, 3 out]
                            n283 = Match Pattern(string=w373, regular expression=":" ("time format string (%c)")) -> (before substring=w378:string)  [unwired: 1 in, 3 out]
                            n284 = Multiply(x=w380, y=60) -> (x*y=w371:i32)
                            n285 = Decimal String To Number(string=w377) -> (number=w372:i32)  [unwired: 2 in, 1 out]
                            n286 = Decimal String To Number(string=w378) -> (number=w370:i32)  [unwired: 2 in, 1 out]
                            n287 = Subtract(x=w371, y=w372) -> (x-y=w369:i32)
                            n288 = Add(x=w369, y=w370) -> (x+y=w368:i32)
                            n289 = Greater Or Equal?(x=5 ("y"), y=w368) -> (x >= y?=w366:bool)
                            n290 = Not(x=w366) -> (.not. x?=w365:bool)
                            n291 = property on="ResetAlarmButton" class="Bool"("Visible"=w365) -> ()  [unwired: 2 in, 2 out]
                          }
                          frame True {
                            n292 = Match Pattern(string=w391, regular expression=":" ("time format string (%c)")) -> (before substring=w388:string)  [unwired: 1 in, 3 out]
                            n293 = Match Pattern(string=w390, regular expression=":" ("time format string (%c)")) -> (before substring=w387:string)  [unwired: 1 in, 3 out]
                            n294 = Decimal String To Number(string=w388) -> (number=w386:i32)  [unwired: 2 in, 1 out]
                            n295 = Decimal String To Number(string=w387) -> (number=w385:i32)  [unwired: 2 in, 1 out]
                            n296 = Subtract(x=w386, y=w385) -> (x-y=w383:i32)
                            n297 = Greater Or Equal?(x=w383, y=5) -> (x >= y?=w382:bool)
                            n298 = Not(x=w382) -> (.not. x?=w381:bool)
                            n299 = property on="ResetAlarmButton" class="Bool"("Visible"=w381) -> ()  [unwired: 2 in, 2 out]
                          }
                        }
                      }
                      frame #2 {
                        n300 = property on="ResetAlarmButton" class="Bool"() -> ("Visible"=w393:bool)  [unwired: 2 in, 2 out]
                        n301 = case shown="False" w393 {
                          frame False {
                            n302 = local read "GeneralParametersArray"() -> (w401:cluster{"Parameter":string, "Value":string}[])
                            n303 = local read "GeneralParametersArray"() -> (w400:cluster{"Parameter":string, "Value":string}[])
                            n304 = local read "GeneralParametersArray"() -> (w406:cluster{"Parameter":string, "Value":string}[])
                            n305 = call "ScanParameters.vi"("MainConfigurationArray"=w401, "Parameter"="LineName") -> ("Value"=w402:string)  [unwired: 9 in]
                            n306 = call "ScanParameters.vi"("MainConfigurationArray"=w400, "Parameter"="SubAssembly") -> ("Value"=w403:string)  [unwired: 9 in]
                            n307 = Concatenate Strings("update \"", w402, "_userlogged\" set \"useroperations\"='0',\"userquality\"='0' where \"subassembly\"='", w403, "'") -> (w404:string)
                            n308 = call "ScanParameters.vi"("MainConfigurationArray"=w406, "Parameter"="ConnectionDSN") -> ("Value"=w407:string)  [unwired: 9 in]
                            n309 = To Lower Case(string=w404) -> (all lower case string=w405:string)
                            n310 = call "SQL_QueryNoReturn.vi"("SQL query"=w405, "ConnectionDSN"=w407) -> ()  [unwired: 10 in]
                          }
                          frame True {
                          }
                        }
                      }
                    }
                  }
                }
              }
              frame #2 {
                w412 = ":" ("regular expression")
                # "Updates de SQL Table with the current values of the counters monitor each minute"
                n311 = local read "Hour"() -> (w414:string)
                n312 = Match Pattern(string=w414, regular expression=w412) -> (after substring=w413:string)  [unwired: 1 in, 3 out]
                n313 = Match Pattern(string=w413, regular expression=w412) -> (after substring=w411:string)  [unwired: 1 in, 3 out]
                n314 = Decimal String To Number(string=w411) -> (number=w410:i32)  [unwired: 2 in, 1 out]
                n315 = Equal?(x=w410, y=1) -> (x = y?=w409:bool)
                n316 = case shown="True" w409 {
                  frame False {
                  }
                  frame True {
                    n317 = stacked-sequence {
                      frame #0 {
                        n318 = local read "GeneralParametersArray"() -> (w424:cluster{"Parameter":string, "Value":string}[])
                        n319 = local read "GeneralParametersArray"() -> (w418:cluster{"Parameter":string, "Value":string}[])
                        n320 = local read "GeneralParametersArray"() -> (w420:cluster{"Parameter":string, "Value":string}[])
                        n321 = local read "Counters Monitor Array"() -> (w415:T16)
                        n322 = call "ScanParameters.vi"("MainConfigurationArray"=w424, "Parameter"="ConnectionDSN") -> ("Value"=w422:string)  [unwired: 9 in]
                        n323 = call "ScanParameters.vi"("MainConfigurationArray"=w418, "Parameter"="SubAssembly") -> ("Value"=w416:string)  [unwired: 9 in]
                        n324 = call "ScanParameters.vi"("MainConfigurationArray"=w420, "Parameter"="LineName") -> ("Value"=w419:string)  [unwired: 9 in]
                        n325 = call "SQL_CountersMonitorUpdate.vi"("Counters Monitor Array"=w415, "SubAssembly"=w416, "LineName"=w419, "ConnectionDSN"=w422) -> ()  [unwired: 8 in]
                      }
                      frame #1 {
                        n326 = local read "CycleTimeArray"() -> (w427:T1)
                        n327 = local read "LastCycleTimePath"() -> (w425:path)
                        n328 = Flatten To JSON(anything=w427) -> (JSON string=w426:string)  [unwired: 2 in, 1 out]
                        n329 = call "SaveParameters.vi"("JSON_Text"=w426, "ShiftConfigPath"=w425) -> ()  [unwired: 10 in]
                      }
                    }
                  }
                }
              }
              frame #3 {
                # "In this frame the plan is to add the check for the configuration enabling in the PLCs\n\n1. it will make a sweep of all the stations and the value of the configuration level enabled in the database, \n      Where\n      0 = Locked\n      1 or grater = Model Change is posible (leader)\n      2 or greater = can view parameters for audit purpose. (quality auditor)\n      3  = can modify the parameters. (engineering/maintenance)"
              }
            }
          }
          event "SavePLCConfig": Value Change {
            n330 = event-data() -> ()  [unwired: 1 in, 6 out]
            n331 = stacked-sequence {
              frame #0 {
                # "Checks if any parameter was changed and stores the changes in the Modification Array to Store modifications in database"
                n332 = local read "PLC Configuration Path"() -> (w436:path)
                n333 = local read "PLC Connection Array"() -> (w433:T11)
                n334 = local read "UserLogged"() -> (w432:string)
                n335 = call "LoadParameters.vi"("ShiftConfigPath"=w436) -> ("JSON_Text"=w435:string)  [unwired: 10 in]
                n336 = Unflatten From JSON(JSON string=w435, type and defaults=w433) -> (value=w434:T11)  [unwired: 5 in, 1 out]
                n337 = Match Pattern(string=w432, regular expression=",") -> (before substring=w430:string)  [unwired: 1 in, 3 out]
                n338 = for {
                  tunnel: w434 -> [w459] mode=indexing
                  tunnel: w433 -> [w458] mode=indexing
                  tunnel: w430 -> [w441]
                  shift-right: [w437] -> w428
                  shift-left: string[] [] -> [w438]
                  # "Before"
                  n339 = Unbundle By Name(w459) -> ("MachineName"=w456:string, "PLC Address"=w455:string, "PLC Type"=w457:u16, "MemoryNumber1"=w453:string, "MemoryNumber2"=w452:string, "MemoryNumber3"=w451:string)
                  n340 = Unbundle By Name(w458) -> ("MachineName"=w450:string, "PLC Address"=w449:string, "PLC Type"=w448:u16, "MemoryNumber1"=w446:string, "MemoryNumber2"=w445:string, "MemoryNumber3"=w444:string)
                  n341 = Number To Decimal String(number=w457) -> (decimal integer string=w454:string)  [unwired: 1 in]
                  n342 = Number To Decimal String(number=w448) -> (decimal integer string=w447:string)  [unwired: 1 in]
                  n343 = Build Array(w456, w455, w454, w453, w452, w451) -> (w440:string[])
                  n344 = Build Array(w450, w449, w447, w446, w445, w444) -> (w439:string[])
                  n345 = Not Equal?(x=w440, y=w439) -> (x != y?=w443:bool[])
                  n346 = Or Array Elements(Boolean array=w443) -> (logical OR=w442:bool)
                  n347 = case shown="True" w442 {
                    tunnel: w441 -> [_ w462]
                    tunnel: w440 -> [_ w464]
                    tunnel: w439 -> [_ w463]
                    tunnel: [w460 w461] -> w437
                    tunnel: w438 -> [w460 w465]
                    frame False {
                    }
                    frame True {
                      n348 = call "SQL_SortModifications.vi"("UserLogged"=w462, "AfterArray"=w463, "BeforeArray"=w464, "CleanArray"=w465) -> ("ResultArray"=w461:string[])  [unwired: 7 in]
                    }
                  }
                }
                n349 = local write "ModificationArray"(w428) -> ()
              }
              frame #1 {
                n350 = Get Date/Time In Seconds() -> (seconds since 1Jan1904=w470:timestamp)
                n351 = local read "UserLogged"() -> (w473:string)
                n352 = local read "ModificationArray"() -> (w474:string[])
                n353 = Format Date/Time String(time format string (%c)="%x", seconds (now)=w470) -> (date/time string=w468:string)  [unwired: 1 in]
                n354 = Format Date/Time String(time format string (%c)="%H:%M:%S", seconds (now)=w470) -> (date/time string=w467:string)  [unwired: 1 in]
                n355 = Match Pattern(string=w473, regular expression=",") -> (before substring=w466:string)  [unwired: 1 in, 3 out]
                n356 = for {
                  tunnel: w474 -> [w478] mode=indexing
                  tunnel: w468 -> [w482]
                  tunnel: w467 -> [w481]
                  tunnel: w466 -> [w480]
                  w479 = "','"
                  n357 = local read "GeneralParametersArray"() -> (w486:cluster{"Parameter":string, "Value":string}[])
                  n358 = local read "GeneralParametersArray"() -> (w490:cluster{"Parameter":string, "Value":string}[])
                  n359 = call "ScanParameters.vi"("MainConfigurationArray"=w486, "Parameter"="LineName") -> ("Value"=w484:string)  [unwired: 9 in]
                  n360 = call "ScanParameters.vi"("MainConfigurationArray"=w490, "Parameter"="ConnectionDSN") -> ("Value"=w488:string)  [unwired: 9 in]
                  n361 = Concatenate Strings("insert into \"", w484, "_systemlog\" values('", w482, w479, w481, w479, w480, w479, w478, "')") -> (w476:string)
                  n362 = To Lower Case(string=w476) -> (all lower case string=w475:string)
                  n363 = call "SQL_QueryNoReturn.vi"("SQL query"=w475, "ConnectionDSN"=w488) -> ()  [unwired: 10 in]
                }
              }
              frame #2 {
                # "Store the PLC Configuration in JSON File"
                n364 = local read "PLC Connection Array"() -> (w502:T11)
                n365 = local read "PLC Configuration Path"() -> (w501:path)
                n366 = Flatten To JSON(anything=w502) -> (JSON string=w500:string)  [unwired: 2 in, 1 out]
                n367 = local read "GeneralParametersArray"() -> (w496:cluster{"Parameter":string, "Value":string}[])
                n368 = local read "GeneralParametersArray"() -> (w492:cluster{"Parameter":string, "Value":string}[])
                n369 = call "SaveParameters.vi"("JSON_Text"=w500, "ShiftConfigPath"=w501) -> ()  [unwired: 10 in]
                n370 = call "ScanParameters.vi"("MainConfigurationArray"=w496, "Parameter"="ConnectionDSN") -> ("Value"=w494:string)  [unwired: 9 in]
                n371 = call "ScanParameters.vi"("MainConfigurationArray"=w492, "Parameter"="LineName") -> ("Value"=w491:string)  [unwired: 9 in]
                n372 = for {
                  tunnel: w502 -> [w506] mode=indexing
                  tunnel: [w503] -> w497 mode=indexing
                  tunnel: w494 -> [w505]
                  tunnel: w491 -> [w504]
                  n373 = Unbundle By Name(w506) -> ("MachineName"=w503:string)
                  n374 = disable-structure shown="Disabled" {
                    disable-tunnel: w505 -> [w510 _]
                    disable-tunnel: w504 -> [w508 _]
                    disable-tunnel: w503 -> [w507 _]
                    frame Disabled {
                      n375 = call "SQL_CycleTime_RegisterMachine.vi"("MachineName"=w507, "LineName"=w508, "TableName"="CycleTime", "ConnectionDSN"=w510) -> ()  [unwired: 8 in]
                    }
                    frame Enabled {
                    }
                  }
                }
                n376 = local read "CounterLineName Path"() -> (w498:path)
                n377 = local read "Line Name"() -> (w499:string)
                n378 = call "SaveParameters.vi"("JSON_Text"=w499, "ShiftConfigPath"=w498) -> ()  [unwired: 10 in]
                n379 = property on="MachineNameID" class="Ring (strict)"("Strings []"=w497) -> ()  [unwired: 2 in, 2 out]
                n380 = property on="Selector_MachineSpareParts" class="Ring (strict)"("Strings []"=w497) -> ()  [unwired: 2 in, 2 out]
              }
            }
          }
          event "SaveCountersConfig": Value Change {
            n381 = event-data() -> ()  [unwired: 1 in, 6 out]
            n382 = stacked-sequence {
              frame #0 {
                n383 = local read "ThisAppPath"() -> (w517:path)
                n384 = local read "MachineNameID"() -> (w523:u16)
                n385 = local read "ModelName"() -> (w515:u16)
                n386 = property on="MachineNameID" class="Ring (strict)"() -> ("Strings []"=w522:string[])  [unwired: 2 in, 2 out]
                n387 = property on="ModelName" class="Ring (strict)"() -> ("Strings []"=w514:string[])  [unwired: 2 in, 2 out]
                n388 = Path To String(path=w517) -> (string=w516:string)
                n389 = Index Array(array=w522, index=w523) -> (element=w520:string)
                n390 = Index Array(array=w514, index=w515) -> (element=w512:string)
                n391 = Concatenate Strings(w516, "\\Config\\CounterSettingConfiguration_" ("regular expression"), w520, "_" ("regular expression"), w512, ".txt" ("regular expression")) -> (w521:string)
                n392 = String To Path(string=w521) -> (path=w519:path)
                n393 = local write "Counters Configuration Path"(w519) -> ()
              }
              frame #1 {
                # "Checks if any parameter was changed and stores the changes in the Modification Array to Store modifications in database"
                n394 = local read "Counters Configuration Path"() -> (w532:path)
                n395 = local read "CountersConfigArray"() -> (w529:T5)
                n396 = local read "UserLogged"() -> (w528:string)
                n397 = call "LoadParameters.vi"("ShiftConfigPath"=w532) -> ("JSON_Text"=w531:string)  [unwired: 10 in]
                n398 = Unflatten From JSON(JSON string=w531, type and defaults=w529) -> (value=w530:T5)  [unwired: 5 in, 1 out]
                n399 = Match Pattern(string=w528, regular expression=",") -> (before substring=w526:string)  [unwired: 1 in, 3 out]
                n400 = for {
                  tunnel: w530 -> [w553] mode=indexing
                  tunnel: w529 -> [w552] mode=indexing
                  tunnel: w526 -> [w541]
                  shift-right: [w537] -> w524
                  shift-left: string[] [] -> [w538]
                  # "Before"
                  n401 = Unbundle By Name(w553) -> ("ToolCribPartNumber"=w550:string, "ComponentName"=w549:string, "PreparationAlarmCounter"=w551:dbl, "StoppageAlarmCounter"=w536:dbl)
                  n402 = Unbundle By Name(w552) -> ("ToolCribPartNumber"=w547:string, "ComponentName"=w546:string, "PreparationAlarmCounter"=w545:dbl, "StoppageAlarmCounter"=w534:dbl)
                  n403 = Number To Decimal String(number=w545) -> (decimal integer string=w544:string)  [unwired: 1 in]
                  n404 = Number To Decimal String(number=w534) -> (decimal integer string=w533:string)  [unwired: 1 in]
                  n405 = Number To Decimal String(number=w551) -> (decimal integer string=w548:string)  [unwired: 1 in]
                  n406 = Number To Decimal String(number=w536) -> (decimal integer string=w535:string)  [unwired: 1 in]
                  n407 = Build Array(w550, w549, w548, w535) -> (w540:string[])
                  n408 = Build Array(w547, w546, w544, w533) -> (w539:string[])
                  n409 = Not Equal?(x=w540, y=w539) -> (x != y?=w543:bool[])
                  n410 = Or Array Elements(Boolean array=w543) -> (logical OR=w542:bool)
                  n411 = case shown="True" w542 {
                    tunnel: w541 -> [_ w556]
                    tunnel: w540 -> [_ w558]
                    tunnel: w539 -> [_ w557]
                    tunnel: [w554 w555] -> w537
                    tunnel: w538 -> [w554 w559]
                    frame False {
                    }
                    frame True {
                      n412 = call "SQL_SortModifications.vi"("UserLogged"=w556, "AfterArray"=w557, "BeforeArray"=w558, "CleanArray"=w559) -> ("ResultArray"=w555:string[])  [unwired: 7 in]
                    }
                  }
                }
                n413 = local write "ModificationArray"(w524) -> ()
              }
              frame #2 {
                n414 = Get Date/Time In Seconds() -> (seconds since 1Jan1904=w564:timestamp)
                n415 = local read "UserLogged"() -> (w567:string)
                n416 = local read "ModificationArray"() -> (w568:string[])
                n417 = Format Date/Time String(time format string (%c)="%x", seconds (now)=w564) -> (date/time string=w562:string)  [unwired: 1 in]
                n418 = Format Date/Time String(time format string (%c)="%H:%M:%S", seconds (now)=w564) -> (date/time string=w561:string)  [unwired: 1 in]
                n419 = Match Pattern(string=w567, regular expression=",") -> (before substring=w560:string)  [unwired: 1 in, 3 out]
                n420 = for {
                  tunnel: w568 -> [w572] mode=indexing
                  tunnel: w562 -> [w576]
                  tunnel: w561 -> [w575]
                  tunnel: w560 -> [w574]
                  w573 = "','"
                  n421 = local read "GeneralParametersArray"() -> (w580:cluster{"Parameter":string, "Value":string}[])
                  n422 = local read "GeneralParametersArray"() -> (w584:cluster{"Parameter":string, "Value":string}[])
                  n423 = call "ScanParameters.vi"("MainConfigurationArray"=w580, "Parameter"="LineName") -> ("Value"=w578:string)  [unwired: 9 in]
                  n424 = call "ScanParameters.vi"("MainConfigurationArray"=w584, "Parameter"="ConnectionDSN") -> ("Value"=w582:string)  [unwired: 9 in]
                  n425 = Concatenate Strings("insert into \"", w578, "_systemlog\" values('", w576, w573, w575, w573, w574, w573, w572, "')") -> (w570:string)
                  n426 = To Lower Case(string=w570) -> (all lower case string=w569:string)
                  n427 = call "SQL_QueryNoReturn.vi"("SQL query"=w569, "ConnectionDSN"=w582) -> ()  [unwired: 10 in]
                }
              }
              frame #3 {
                n428 = local read "CountersConfigArray"() -> (w586:T5)
                n429 = local read "Counters Configuration Path"() -> (w585:path)
                n430 = Flatten To JSON(anything=w586) -> (JSON string=w587:string)  [unwired: 2 in, 1 out]
                n431 = call "SaveParameters.vi"("JSON_Text"=w587, "ShiftConfigPath"=w585) -> ()  [unwired: 10 in]
              }
            }
          }
          event "SaveCurrentCounter": Value Change {
            n432 = event-data() -> ()  [unwired: 1 in, 6 out]
            n433 = local read "Counters Monitor Array"() -> (w588:T16)
            n434 = local read "CurrentCountersPath"() -> (w590:path)
            n435 = Flatten To JSON(anything=w588) -> (JSON string=w589:string)  [unwired: 2 in, 1 out]
            n436 = call "SaveParameters.vi"("JSON_Text"=w589, "ShiftConfigPath"=w590) -> ()  [unwired: 10 in]
          }
          event "SaveGeneralConfig": Value Change {
            n437 = event-data() -> ()  [unwired: 1 in, 6 out]
            n438 = stacked-sequence {
              frame #0 {
                # "Checks if any parameter was changed and stores the changes in the Modification Array to Store modifications in database"
                n439 = local read "GeneralParametersArray"() -> (w596:cluster{"Parameter":string, "Value":string}[])
                n440 = local read "GeneralConfigPath"() -> (w599:path)
                n441 = local read "UserLogged"() -> (w595:string)
                n442 = call "LoadParameters.vi"("ShiftConfigPath"=w599) -> ("JSON_Text"=w598:string)  [unwired: 10 in]
                n443 = Unflatten From JSON(JSON string=w598, type and defaults=w596) -> (value=w597:cluster{"Parameter":string, "Value":string}[])  [unwired: 5 in, 1 out]
                n444 = Match Pattern(string=w595, regular expression=",") -> (before substring=w593:string)  [unwired: 1 in, 3 out]
                n445 = for {
                  tunnel: w597 -> [w612] mode=indexing
                  tunnel: w596 -> [w611] mode=indexing
                  tunnel: w593 -> [w604]
                  shift-right: [w600] -> w591
                  shift-left: string[] [] -> [w601]
                  # "Before"
                  n446 = Unbundle By Name(w611) -> ("Parameter"=w608:string, "Value"=w607:string)
                  n447 = Unbundle By Name(w612) -> ("Parameter"=w610:string, "Value"=w609:string)
                  n448 = Build Array(w610, w609) -> (w603:string[])
                  n449 = Build Array(w608, w607) -> (w602:string[])
                  n450 = Not Equal?(x=w603, y=w602) -> (x != y?=w606:bool[])
                  n451 = Or Array Elements(Boolean array=w606) -> (logical OR=w605:bool)
                  n452 = case shown="True" w605 {
                    tunnel: w604 -> [_ w615]
                    tunnel: w603 -> [_ w617]
                    tunnel: w602 -> [_ w616]
                    tunnel: [w613 w614] -> w600
                    tunnel: w601 -> [w613 w618]
                    frame False {
                    }
                    frame True {
                      n453 = call "SQL_SortModifications.vi"("UserLogged"=w615, "AfterArray"=w616, "BeforeArray"=w617, "CleanArray"=w618) -> ("ResultArray"=w614:string[])  [unwired: 7 in]
                    }
                  }
                }
                n454 = local write "ModificationArray"(w591) -> ()
              }
              frame #1 {
                n455 = Get Date/Time In Seconds() -> (seconds since 1Jan1904=w623:timestamp)
                n456 = local read "UserLogged"() -> (w626:string)
                n457 = local read "ModificationArray"() -> (w627:string[])
                n458 = Format Date/Time String(time format string (%c)="%x", seconds (now)=w623) -> (date/time string=w621:string)  [unwired: 1 in]
                n459 = Format Date/Time String(time format string (%c)="%H:%M:%S", seconds (now)=w623) -> (date/time string=w620:string)  [unwired: 1 in]
                n460 = Match Pattern(string=w626, regular expression=",") -> (before substring=w619:string)  [unwired: 1 in, 3 out]
                n461 = for {
                  tunnel: w627 -> [w631] mode=indexing
                  tunnel: w621 -> [w635]
                  tunnel: w620 -> [w634]
                  tunnel: w619 -> [w633]
                  w632 = "','"
                  n462 = local read "GeneralParametersArray"() -> (w639:cluster{"Parameter":string, "Value":string}[])
                  n463 = local read "GeneralParametersArray"() -> (w643:cluster{"Parameter":string, "Value":string}[])
                  n464 = call "ScanParameters.vi"("MainConfigurationArray"=w639, "Parameter"="LineName") -> ("Value"=w637:string)  [unwired: 9 in]
                  n465 = call "ScanParameters.vi"("MainConfigurationArray"=w643, "Parameter"="ConnectionDSN") -> ("Value"=w641:string)  [unwired: 9 in]
                  n466 = Concatenate Strings("insert into \"", w637, "_systemlog\" values('", w635, w632, w634, w632, w633, w632, w631, "')") -> (w629:string)
                  n467 = To Lower Case(string=w629) -> (all lower case string=w628:string)
                  n468 = call "SQL_QueryNoReturn.vi"("SQL query"=w628, "ConnectionDSN"=w641) -> ()  [unwired: 10 in]
                }
              }
              frame #2 {
                n469 = local read "GeneralParametersArray"() -> (w644:cluster{"Parameter":string, "Value":string}[])
                n470 = local read "GeneralConfigPath"() -> (w646:path)
                n471 = Flatten To JSON(anything=w644) -> (JSON string=w645:string)  [unwired: 2 in, 1 out]
                n472 = call "SaveParameters.vi"("JSON_Text"=w645, "ShiftConfigPath"=w646) -> ()  [unwired: 10 in]
              }
              frame #3 {
                n473 = local read "GeneralParametersArray"() -> (w647:cluster{"Parameter":string, "Value":string}[])
                n474 = for {
                  tunnel: w647 -> [w648] mode=indexing
                  n475 = Unbundle By Name(w648) -> ()  [unwired: 2 out]
                }
              }
              frame #4 {
                n476 = local read "GeneralParametersArray"() -> (w655:cluster{"Parameter":string, "Value":string}[])
                n477 = call "ScanParameters.vi"("MainConfigurationArray"=w655, "Parameter"="Models") -> ("Value"=w650:string)  [unwired: 9 in]
                n478 = Spreadsheet String To Array(delimiter (Tab)=",", format string="%s" ("spreadsheet string"), spreadsheet string=w650, array type (2D Dbl)=string[] []) -> (array=w649:string[])
                n479 = property on="ModelName" class="Ring (strict)"("Strings []"=w649) -> ()  [unwired: 2 in, 2 out]
              }
            }
          }
          event "SaveDictionary": Value Change {
            n480 = event-data() -> ()  [unwired: 1 in, 6 out]
            n481 = local read "DictionaryArray"() -> (w658:T14)
            n482 = local read "PathDictionary"() -> (w656:path)
            n483 = Flatten To JSON(anything=w658) -> (JSON string=w657:string)  [unwired: 2 in, 1 out]
            n484 = call "SaveParameters.vi"("JSON_Text"=w657, "ShiftConfigPath"=w656) -> ()  [unwired: 10 in]
          }
          event "RefreshCountersConfig": Value Change {
            n485 = event-data() -> ()  [unwired: 1 in, 6 out]
            n486 = local read "MachineNameID"() -> (w668:u16)
            n487 = local read "ThisAppPath"() -> (w660:path)
            n488 = property on="MachineNameID" class="Ring (strict)"() -> ("Strings []"=w667:string[])  [unwired: 2 in, 2 out]
            n489 = Path To String(path=w660) -> (string=w659:string)
            n490 = Index Array(array=w667, index=w668) -> (element=w665:string)
            n491 = Concatenate Strings(w659, "\\Config\\CounterSettingConfiguration_" ("regular expression"), w665, ".txt" ("regular expression")) -> (w666:string)
            n492 = String To Path(string=w666) -> (path=w661:path)
            n493 = call <vilib>:"Check if File or Folder Exists.vi"("path"=w661) -> ("file or folder exists?"=w662:bool)  [unwired: 8 in, 2 out]
            n494 = case shown="True" w662 {
              tunnel: w661 -> [_ w672]
              frame False {
                n495 = local write "CountersConfigArray"(T5 [] ("CountersConfigArray")) -> ()
              }
              frame True {
                n496 = local read "CountersConfigArray"() -> (w671:T5)
                n497 = call "LoadParameters.vi"("ShiftConfigPath"=w672) -> ("JSON_Text"=w673:string)  [unwired: 10 in]
                n498 = local write "Counters Configuration Path"(w672) -> ()
                n499 = Unflatten From JSON(JSON string=w673, type and defaults=w671) -> (value=w670:T5)  [unwired: 5 in, 1 out]
                n500 = local write "CountersConfigArray"(w670) -> ()
              }
            }
          }
          event "RefreshPLCConfig": Value Change {
            # "Load PLC Connection Information"
            n501 = event-data() -> ()  [unwired: 1 in, 6 out]
            n502 = local read "PLC Configuration Path"() -> (w675:path)
            n503 = local read "PLC Connection Array"() -> (w676:T11)
            n504 = call "LoadParameters.vi"("ShiftConfigPath"=w675) -> ("JSON_Text"=w674:string)  [unwired: 10 in]
            n505 = Unflatten From JSON(JSON string=w674, type and defaults=w676) -> (value=w677:T11)  [unwired: 5 in, 1 out]
            n506 = local write "PLC Connection Array"(w677) -> ()
          }
          event "RefreshGeneralConfig": Value Change {
            n507 = event-data() -> ()  [unwired: 1 in, 6 out]
            n508 = stacked-sequence {
              frame #0 {
                n509 = local read "GeneralConfigPath"() -> (w681:path)
                n510 = local read "GeneralParametersArray"() -> (w679:cluster{"Parameter":string, "Value":string}[])
                n511 = call "LoadParameters.vi"("ShiftConfigPath"=w681) -> ("JSON_Text"=w680:string)  [unwired: 10 in]
                n512 = Unflatten From JSON(JSON string=w680, type and defaults=w679) -> (value=w678:cluster{"Parameter":string, "Value":string}[])  [unwired: 5 in, 1 out]
                n513 = local write "GeneralParametersArray"(w678) -> ()
              }
              frame #1 {
                n514 = local read "GeneralParametersArray"() -> (w683:cluster{"Parameter":string, "Value":string}[])
                n515 = call "ScanParameters.vi"("MainConfigurationArray"=w683, "Parameter"="LineName") -> ("Value"=w684:string)  [unwired: 9 in]
                n516 = local write "Line Name"(w684) -> ()
              }
            }
          }
          event "RefreshCurrentCounter": Value Change {
            n517 = event-data() -> ()  [unwired: 1 in, 6 out]
            n518 = local read "CurrentCountersPath"() -> (w688:path)
            n519 = local read "Counters Monitor Array"() -> (w686:T16)
            n520 = call "LoadParameters.vi"("ShiftConfigPath"=w688) -> ("JSON_Text"=w687:string)  [unwired: 10 in]
            n521 = Unflatten From JSON(JSON string=w687, type and defaults=w686) -> (value=w685:T16)  [unwired: 5 in, 1 out]
            n522 = local write "Counters Monitor Array"(w685) -> ()
          }
          event "ResetAlarm": Value Change {
            n523 = event-data() -> ()  [unwired: 1 in, 6 out]
            n524 = local read "Counters Monitor Array"() -> (w690:T16)
            n525 = local read "ResetAlarm"() -> (w693:bool[])
            n526 = local read "ArrayAlarm"() -> (w692:bool[])
            n527 = for {
              tunnel: w693 -> [w699] mode=indexing
              tunnel: w692 -> [w696] mode=indexing
              tunnel: [w697] -> w691 mode=indexing
              tunnel: w690 -> [w694] mode=indexing
              tunnel: [w695] -> w689 mode=indexing
              n528 = And(x=w699, y=w696) -> (x .and. y?=w698:bool)
              n529 = case shown="True" w698 {
                tunnel: [w701 FALSE] -> w697
                tunnel: w696 -> [w701 _]
                tunnel: w694 -> [w700 _]
                tunnel: [w700 w705] -> w695
                tunnel: w694 -> [_ w703]
                frame False {
                }
                frame True {
                  n530 = local read "OnlineStations"() -> (w702:T15)
                  n531 = Unbundle By Name(w703) -> ("MachineName"=w704:string)
                  n532 = Bundle By Name(cluster=w703, "CurrentCount"=0) -> (w705:T18)
                  n533 = for {
                    tunnel: w704 -> [w713]
                    tunnel: w702 -> [w715] mode=indexing
                    n534 = Unbundle By Name(w715) -> ("MachineName"=w714:string, "Connection"=w712:bool)
                    n535 = Equal?(x=w712, y=TRUE) -> (x = y?=w710:bool)
                    n536 = Equal?(x=w713, y=w714) -> (x = y?=w709:bool)
                    n537 = And(x=w709, y=w710) -> (x .and. y?=w708:bool)
                    n538 = case shown="True" w708 {
                      tunnel: w713 -> [_ w717]
                      frame False {
                      }
                      frame True {
                        (unwired) 0
                        # "Reset the alarm in the PLC"
                        n539 = local read "PLC Connection Array"() -> (w720:T11)
                        n540 = for {
                          tunnel: w720 -> [w729] mode=indexing
                          tunnel: w717 -> [w727]
                          shift-right: [w724] -> w721
                          shift-left: "" -> [w723]
                          tunnel: [w722] -> w716
                          n541 = Unbundle By Name(w729) -> ("MachineName"=w728:string, "PLC Address"=w725:string, "MemoryNumber2"=w722:string)
                          n542 = Equal?(x=w727, y=w728) -> (x = y?=w726:bool)
                          n543 = case shown="False" w726 {
                            tunnel: w725 -> [_ w731]
                            tunnel: [w730 w731] -> w724
                            tunnel: w723 -> [w730 _]
                            frame False {
                            }
                            frame True {
                            }
                          }
                        }
                        n544 = call "CBM_WriteBool_PLC_Keyence.vi"("Set?"=FALSE, "MemoryNumber"=w716, "PLC_IP"=w721) -> ()  [unwired: 8 in, 1 out]
                      }
                    }
                  }
                }
              }
            }
            n545 = local write "Counters Monitor Array"(w689) -> ()
            n546 = local write "ArrayAlarm"(w691) -> ()
          }
          event "RefreshLists": Value Change {
            # "Load PLC Connection Information"
            n547 = event-data() -> ()  [unwired: 1 in, 6 out]
            n548 = local read "PLC Configuration Path"() -> (w734:path)
            n549 = local read "PLC Connection Array"() -> (w735:T11)
            n550 = call "LoadParameters.vi"("ShiftConfigPath"=w734) -> ("JSON_Text"=w733:string)  [unwired: 10 in]
            n551 = Unflatten From JSON(JSON string=w733, type and defaults=w735) -> (value=w732:T11)  [unwired: 5 in, 1 out]
            n552 = local write "PLC Connection Array"(w732) -> ()
            n553 = for {
              tunnel: w732 -> [w737] mode=indexing
              tunnel: [w738] -> w736 mode=indexing
              n554 = Unbundle By Name(w737) -> ("MachineName"=w738:string)
            }
            n555 = property on="Selector_MachineSpareParts" class="Ring (strict)"("Strings []"=w736) -> ()  [unwired: 2 in, 2 out]
          }
          event "ResetAlarmButton": Value Change {
            n556 = event-data() -> ()  [unwired: 1 in, 6 out]
            n557 = local read "GeneralParametersArray"() -> (w742:cluster{"Parameter":string, "Value":string}[])
            n558 = local read "GeneralParametersArray"() -> (w745:cluster{"Parameter":string, "Value":string}[])
            n559 = local read "Counters Monitor Array"() -> (w749:T16)
            n560 = local read "PLC Connection Array"() -> (w739:T11)
            n561 = local read "OnlineStations"() -> (w750:T15)
            n562 = local read "ArrayAlarm"() -> (w746:bool[])
            n563 = call "ScanParameters.vi"("MainConfigurationArray"=w742, "Parameter"="LineName") -> ("Value"=w740:string)  [unwired: 9 in]
            n564 = call "ScanParameters.vi"("MainConfigurationArray"=w745, "Parameter"="ConnectionDSN") -> ("Value"=w743:string)  [unwired: 9 in]
            n565 = call "ResetAlarm.vi"("LineName"=w740, "ConnectionDSN"=w743, "ArrayAlarmIN"=w746, "PLC Connection Array"=w739, "OnlineStations"=w750, "Counters Monitor Array IN"=w749) -> ("ArrayAlarmOUT"=w747:bool[], "Counters Monitor Array OUT"=w748:T16)  [unwired: 4 in]
            n566 = local write "Counters Monitor Array"(w748) -> ()
            n567 = local write "ArrayAlarm"(w747) -> ()
          }
          event "MachineNameID": Value Change {
            n568 = event-data() -> ()  [unwired: 1 in, 6 out]
            n569 = local read "ThisAppPath"() -> (w759:path)
            n570 = local read "MachineNameID"() -> (w762:u16)
            n571 = local read "ModelName"() -> (w757:u16)
            n572 = property on="MachineNameID" class="Ring (strict)"() -> ("Strings []"=w761:string[])  [unwired: 2 in, 2 out]
            n573 = property on="ModelName" class="Ring (strict)"() -> ("Strings []"=w756:string[])  [unwired: 2 in, 2 out]
            n574 = Path To String(path=w759) -> (string=w758:string)
            n575 = Index Array(array=w761, index=w762) -> (element=w760:string)
            n576 = Index Array(array=w756, index=w757) -> (element=w755:string)
            n577 = Concatenate Strings(w758, "\\Config\\CounterSettingConfiguration_" ("regular expression"), w760, "_" ("regular expression"), w755, ".txt" ("regular expression")) -> (w751:string)
            n578 = String To Path(string=w751) -> (path=w763:path)
            n579 = call <vilib>:"Check if File or Folder Exists.vi"("path"=w763) -> ("file or folder exists?"=w764:bool)  [unwired: 8 in, 2 out]
            n580 = case shown="True" w764 {
              tunnel: w763 -> [_ w768]
              frame False {
                n581 = local write "CountersConfigArray"(T5 [] ("CountersConfigArray")) -> ()
              }
              frame True {
                n582 = local read "CountersConfigArray"() -> (w766:T5)
                n583 = call "LoadParameters.vi"("ShiftConfigPath"=w768) -> ("JSON_Text"=w769:string)  [unwired: 10 in]
                n584 = local write "Counters Configuration Path"(w768) -> ()
                n585 = Unflatten From JSON(JSON string=w769, type and defaults=w766) -> (value=w767:T5)  [unwired: 5 in, 1 out]
                n586 = local write "CountersConfigArray"(w767) -> ()
              }
            }
          }
          event "ModelName": Value Change {
            n587 = event-data() -> ()  [unwired: 1 in, 6 out]
            n588 = local read "ThisAppPath"() -> (w778:path)
            n589 = local read "MachineNameID"() -> (w781:u16)
            n590 = local read "ModelName"() -> (w776:u16)
            n591 = property on="MachineNameID" class="Ring (strict)"() -> ("Strings []"=w780:string[])  [unwired: 2 in, 2 out]
            n592 = property on="ModelName" class="Ring (strict)"() -> ("Strings []"=w775:string[])  [unwired: 2 in, 2 out]
            n593 = Path To String(path=w778) -> (string=w777:string)
            n594 = Index Array(array=w780, index=w781) -> (element=w779:string)
            n595 = Index Array(array=w775, index=w776) -> (element=w774:string)
            n596 = Concatenate Strings(w777, "\\Config\\CounterSettingConfiguration_" ("regular expression"), w779, "_" ("regular expression"), w774, ".txt" ("regular expression")) -> (w773:string)
            n597 = String To Path(string=w773) -> (path=w782:path)
            n598 = call <vilib>:"Check if File or Folder Exists.vi"("path"=w782) -> ("file or folder exists?"=w783:bool)  [unwired: 8 in, 2 out]
            n599 = case shown="True" w783 {
              tunnel: w782 -> [_ w787]
              frame False {
                n600 = local write "CountersConfigArray"(T5 [] ("CountersConfigArray")) -> ()
              }
              frame True {
                n601 = local read "CountersConfigArray"() -> (w785:T5)
                n602 = call "LoadParameters.vi"("ShiftConfigPath"=w787) -> ("JSON_Text"=w788:string)  [unwired: 10 in]
                n603 = local write "Counters Configuration Path"(w787) -> ()
                n604 = Unflatten From JSON(JSON string=w788, type and defaults=w785) -> (value=w786:T5)  [unwired: 5 in, 1 out]
                n605 = local write "CountersConfigArray"(w786) -> ()
              }
            }
          }
          event "Count Signal": Value Change {
            n606 = event-data() -> ()  [unwired: 1 in, 6 out]
            n607 = local read "OnlineStations"() -> (w789:T15)
            n608 = local read "Count Signal"() -> (w790:bool[])
            n609 = for {
              tunnel: w790 -> [w792] mode=indexing
              tunnel: w789 -> [w793] mode=indexing
              n610 = Unbundle By Name(w793) -> ("MachineName"=w791:string)
              n611 = case shown="True" w792 {
                tunnel: w791 -> [_ w795]
                frame False {
                }
                frame True {
                  n612 = local read "Counters Monitor Array"() -> (w796:T16)
                  n613 = for {
                    tunnel: w796 -> [w799] mode=indexing
                    tunnel: w795 -> [w802]
                    tunnel: [w797] -> w794 mode=indexing
                    n614 = Unbundle By Name(w799) -> ("MachineName"=w803:string, "CurrentCount"=w800:i32)
                    n615 = Equal?(x=w802, y=w803) -> (x = y?=w801:bool)
                    n616 = case shown="False" w801 {
                      tunnel: w800 -> [w804 w806]
                      tunnel: [w804 w805] -> w798
                      frame False {
                      }
                      frame True {
                        n617 = Increment(x=w806) -> (x+1=w805:i32)
                      }
                    }
                    n618 = Bundle By Name(cluster=w799, "CurrentCount"=w798) -> (w797:T18)
                  }
                  n619 = local write "Counters Monitor Array"(w794) -> ()
                }
              }
            }
          }
          event "Sort": Value Change {
            n620 = event-data() -> ()  [unwired: 1 in, 6 out]
            n621 = local read "Counters Monitor Array"() -> (w816:T16)
            n622 = for {
              tunnel: w816 -> [w826] mode=indexing
              tunnel: [w825] -> w814 mode=indexing
              tunnel: [w824] -> w813 mode=indexing
              tunnel: [w822] -> w812 mode=indexing
              tunnel: [w820] -> w811 mode=indexing
              tunnel: [w818] -> w810 mode=indexing
              tunnel: [w817] -> w809 mode=indexing
              n623 = Unbundle By Name(w826) -> ("MachineName"=w825:string, "ComponentName"=w824:string, "StoppageAlarmCounter"=w823:i32, "CurrentCount"=w821:i32, "StatusColorBox"=w819:u32, "ToolCribPartNumber"=w817:string)
              n624 = Number To Decimal String(number=w819) -> (decimal integer string=w818:string)  [unwired: 1 in]
              n625 = Number To Decimal String(number=w823) -> (decimal integer string=w822:string)  [unwired: 1 in]
              n626 = Number To Decimal String(number=w821) -> (decimal integer string=w820:string)  [unwired: 1 in]
            }
            n627 = property on="Table Control" class="Tbl (strict)"("Column Headers[]"=string[] ["MachineName", "ComponentName", "StoppageCounter", "CurrentCount", "StatusColorBox", "ToolCribPartNumber"]) -> ()  [unwired: 2 in, 2 out]
            n628 = Build Array(w814, w813, w812, w811, w810, w809) -> (w808:string[][])
            n629 = Transpose 2D Array(2D array=w808) -> (transposed array=w807:string[][])
            n630 = local write "Table Control"(w807) -> ()
          }
          event "Selector_MachineSpareParts": Value Change {
            n631 = event-data() -> ()  [unwired: 1 in, 6 out]
            n632 = local read "Selector_MachineSpareParts"() -> (w836:u16)
            n633 = property on="Selector_MachineSpareParts" class="Ring (strict)"() -> ("Strings []"=w829:string[])  [unwired: 2 in, 2 out]
            n634 = local read "ThisAppPath"() -> (w828:path)
            n635 = Index Array(array=w829, index=w836) -> (element=w834:string)
            n636 = Path To String(path=w828) -> (string=w827:string)
            n637 = Concatenate Strings(w827, "\\Config\\CounterSettingConfiguration_" ("regular expression"), w834, ".txt" ("regular expression")) -> (w835:string)
            n638 = String To Path(string=w835) -> (path=w832:path)
            n639 = call <vilib>:"Check if File or Folder Exists.vi"("path"=w832) -> ("file or folder exists?"=w833:bool)  [unwired: 8 in, 2 out]
            n640 = case shown="True" w833 {
              tunnel: w832 -> [_ w841]
              frame False {
                n641 = local write "CountersConfigArray"(T5 [] ("CountersConfigArray")) -> ()
              }
              frame True {
                n642 = local read "CountersConfigArray"() -> (w840:T5)
                n643 = call "LoadParameters.vi"("ShiftConfigPath"=w841) -> ("JSON_Text"=w842:string)  [unwired: 10 in]
                n644 = Unflatten From JSON(JSON string=w842, type and defaults=w840) -> (value=w838:T5)  [unwired: 5 in, 1 out]
                n645 = for {
                  tunnel: [w845] -> w839 mode=indexing
                  tunnel: w838 -> [w843] mode=indexing
                  n646 = Unbundle By Name(w843) -> ("ToolCribPartNumber"=w848:string, "ComponentName"=w846:string)
                  n647 = call <vilib>:"Space Constant.vi"() -> ("String"=w844:string)
                  n648 = Concatenate Strings(w848, w844, "-", w844, w846) -> (w845:string)
                }
                n649 = property on="Selector_P#-Description" class="Ring (strict)"("Strings []"=w839) -> ()  [unwired: 2 in, 2 out]
              }
            }
          }
          event "Selector_P#-Description": Value Change {
            n650 = event-data() -> ()  [unwired: 1 in, 6 out]
            n651 = stacked-sequence {
              frame #0 {
                w852 = "_"
                n652 = local read "Selector_MachineSpareParts"() -> (w867:u16)
                n653 = local read "Selector_P#-Description"() -> (w865:u16)
                n654 = property on="Selector_MachineSpareParts" class="Ring (strict)"() -> ("Strings []"=w866:string[])  [unwired: 2 in, 2 out]
                n655 = property on="Selector_P#-Description" class="Ring (strict)"() -> ("Strings []"=w864:string[])  [unwired: 2 in, 2 out]
                n656 = local read "ThisAppPath"() -> (w849:path)
                n657 = Index Array(array=w866, index=w867) -> (element=w860:string)
                n658 = Path To String(path=w849) -> (string=w850:string)
                n659 = Index Array(array=w864, index=w865) -> (element=w857:string)
                n660 = call <vilib>:"Space Constant.vi"() -> ("String"=w856:string)
                n661 = Concatenate Strings(w850, "\\Photos\\Spare Parts\\" ("regular expression")) -> (w858:string)
                n662 = Search and Replace String(input string=w857, search string=w856, replace string="") -> (result string=w854:string)  [unwired: 5 in, 3 out]
                n663 = Search and Replace String(input string=w854, search string="-", replace string=w852) -> (result string=w851:string)  [unwired: 5 in, 3 out]
                n664 = Concatenate Strings(w858, w860, w852, w851, ".jpg") -> (w862:string)
                n665 = String To Path(string=w862) -> (path=w861:path)
                n666 = local write "PathSparePartImage"(w861) -> ()
              }
              frame #1 {
                w871 = "_"
                n667 = local read "Selector_MachineSpareParts"() -> (w886:u16)
                n668 = local read "Selector_P#-Description"() -> (w884:u16)
                n669 = property on="Selector_MachineSpareParts" class="Ring (strict)"() -> ("Strings []"=w885:string[])  [unwired: 2 in, 2 out]
                n670 = property on="Selector_P#-Description" class="Ring (strict)"() -> ("Strings []"=w883:string[])  [unwired: 2 in, 2 out]
                n671 = local read "ThisAppPath"() -> (w869:path)
                n672 = Path To String(path=w869) -> (string=w868:string)
                n673 = Index Array(array=w885, index=w886) -> (element=w879:string)
                n674 = Index Array(array=w883, index=w884) -> (element=w876:string)
                n675 = call <vilib>:"Space Constant.vi"() -> ("String"=w875:string)
                n676 = Concatenate Strings(w868, "\\Photos\\Machine Location\\" ("regular expression")) -> (w877:string)
                n677 = Search and Replace String(input string=w876, search string=w875, replace string="") -> (result string=w873:string)  [unwired: 5 in, 3 out]
                n678 = Search and Replace String(input string=w873, search string="-", replace string=w871) -> (result string=w870:string)  [unwired: 5 in, 3 out]
                n679 = Concatenate Strings(w877, w879, w871, w870, ".jpg") -> (w881:string)
                n680 = String To Path(string=w881) -> (path=w880:path)
                n681 = local write "PathLocationMachineImage"(w880) -> ()
              }
              frame #2 {
                n682 = local read "PathLocationMachineImage"() -> (w887:path)
                n683 = local read "PathSparePartImage"() -> (w890:path)
                n684 = call <vilib>:"Check if File or Folder Exists.vi"("path"=w887) -> ("file or folder exists?"=w888:bool)  [unwired: 8 in, 2 out]
                n685 = call <vilib>:"Check if File or Folder Exists.vi"("path"=w890) -> ("file or folder exists?"=w889:bool)  [unwired: 8 in, 2 out]
                n686 = case shown="True" w888 {
                  tunnel: w887 -> [w891 w899]
                  frame False {
                    n687 = Path To String(path=w891) -> (string=w896:string)
                    n688 = Concatenate Strings("La imagen " ("string"), w896, " no existe." ("string")) -> (w895:string)
                    n689 = One Button Dialog(message=w895, button name ("OK")="OK" ("string")) -> ()  [unwired: 1 out]
                  }
                  frame True {
                    w897 = T20 4 items=["Grayscale (U8)", "Grayscale (I16)", "Grayscale (SGL)", "Complex (CSG)", "RGB (U32)", "HSL (U32)", "RGB (U64)", "Grayscale (U16)"] ("Image Type")
                    n690 = call "IMAQ Create"("Image Name"="LocationInMachine", "Image Type"=w897) -> ("New Image"=w901:T10)  [unwired: 3 in, 1 out]
                    n691 = call "IMAQ ReadFile"("File Path"=w899, "Load Color Palette? (No)"=TRUE, "Image"=w901) -> ("Image Out"=w900:T10)  [unwired: 4 in, 4 out]
                    n692 = local write "Image_LocationInMachine"(w900) -> ()
                  }
                }
                n693 = case shown="True" w889 {
                  tunnel: w890 -> [w907 w914]
                  frame False {
                    n694 = Path To String(path=w907) -> (string=w906:string)
                    n695 = Concatenate Strings("La imagen " ("string"), w906, " no existe." ("string")) -> (w904:string)
                    n696 = One Button Dialog(message=w904, button name ("OK")="OK" ("string")) -> ()  [unwired: 1 out]
                  }
                  frame True {
                    w909 = T20 4 items=["Grayscale (U8)", "Grayscale (I16)", "Grayscale (SGL)", "Complex (CSG)", "RGB (U32)", "HSL (U32)", "RGB (U64)", "Grayscale (U16)"] ("Image Type")
                    n697 = call "IMAQ Create"("Image Name"="SparePart", "Image Type"=w909) -> ("New Image"=w912:T10)  [unwired: 3 in, 1 out]
                    n698 = call "IMAQ ReadFile"("File Path"=w914, "Load Color Palette? (No)"=TRUE, "Image"=w912) -> ("Image Out"=w913:T10)  [unwired: 4 in, 4 out]
                    n699 = local write "Image_SparePart"(w913) -> ()
                  }
                }
              }
            }
          }
          event "GDrive": Value Change {
            n700 = event-data() -> ()  [unwired: 1 in, 6 out]
          }
          event "AddUser": Value Change {
            n701 = event-data() -> ()  [unwired: 1 in, 6 out]
            n702 = local read "GeneralParametersArray"() -> (w920:cluster{"Parameter":string, "Value":string}[])
            n703 = local read "GeneralParametersArray"() -> (w917:cluster{"Parameter":string, "Value":string}[])
            n704 = call "ScanParameters.vi"("MainConfigurationArray"=w920, "Parameter"="ConnectionDSN") -> ("Value"=w916:string)  [unwired: 9 in]
            n705 = call "ScanParameters.vi"("MainConfigurationArray"=w917, "Parameter"="UsersTable") -> ("Value"=w915:string)  [unwired: 9 in]
            n706 = call "SQL_CreateUser.vi"("UsersTable"=w915, "ConnectionDSN"=w916) -> ()  [unwired: 10 in]
          }
          event "RefreshDictionary": Value Change {
            n707 = event-data() -> ()  [unwired: 1 in, 6 out]
            n708 = local read "PathDictionary"() -> (w921:path)
            n709 = call <vilib>:"Check if File or Folder Exists.vi"("path"=w921) -> ("file or folder exists?"=w922:bool)  [unwired: 8 in, 2 out]
            n710 = case shown="True" w922 {
              tunnel: w921 -> [_ w925]
              frame False {
              }
              frame True {
                n711 = local read "DictionaryArray"() -> (w926:T14)
                n712 = call "LoadParameters.vi"("ShiftConfigPath"=w925) -> ("JSON_Text"=w924:string)  [unwired: 10 in]
                n713 = Unflatten From JSON(JSON string=w924, type and defaults=w926) -> (value=w923:T14)  [unwired: 5 in, 1 out]
                n714 = local write "DictionaryArray"(w923) -> ()
              }
            }
          }
          event "Login": Value Change {
            w927 = T19."Disabled and Grayed Out" ("Disabled")
            n715 = event-data() -> ()  [unwired: 1 in, 6 out]
            n716 = local read "GeneralParametersArray"() -> (w935:cluster{"Parameter":string, "Value":string}[])
            n717 = local read "GeneralParametersArray"() -> (w934:cluster{"Parameter":string, "Value":string}[])
            n718 = call "ScanParameters.vi"("MainConfigurationArray"=w935, "Parameter"="ConnectionDSN") -> ("Value"=w931:string)  [unwired: 9 in]
            n719 = call "ScanParameters.vi"("MainConfigurationArray"=w934, "Parameter"="UsersTable") -> ("Value"=w930:string)  [unwired: 9 in]
            n720 = property on="PLC Connection Array" class="Arr (strict)"("DisabledEnum"=w927) -> ()  [unwired: 2 in, 2 out]
            n721 = property on="CountersConfigArray" class="Arr (strict)"("DisabledEnum"=w927) -> ()  [unwired: 2 in, 2 out]
            n722 = call "SQL_Login.vi"("UsersTable"=w930, "ConnectionDSN"=w931) -> ("qLevel"=w928:i32, "User"=w929:string)  [unwired: 8 in]
            n723 = local write "UserLevel"(w928) -> ()
            n724 = local write "UserLogged"(w929) -> ()
          }
          event "ShowParetto": Value Change {
            n725 = event-data() -> ()  [unwired: 1 in, 6 out]
          }
          event "LoadDefaultConfig": Value Change {
            n726 = event-data() -> ()  [unwired: 1 in, 6 out]
            n727 = local write "GeneralParametersArray"(cluster{"Parameter":string, "Value":string}[] [{"Parameter"="SenderMail", "Value"="maintenance.nidec.bermudez@gmail.com"}, {"Parameter"="Password", "Value"="Nidec123"}, {"Parameter"="IncidenceRecipients", "Value"="edgar.cruz@nidec.com"}, {"Parameter"="LineName", "Value"="EPSL3"}, {"Parameter"="ConnectionDSN", "Value"="PostgreSQL30"}, {"Parameter"="UsersTable", "Value"="Users"}, {"Parameter"="NidecServer", "Value"="10.110.3.23"}, {"Parameter"="EmailsEnabled", "Value"="Disabled"}] ("GeneralParametersArray")) -> ()
          }
          event "Logout": Value Change {
            w952 = T19."Disabled and Grayed Out" ("Disabled")
            n728 = event-data() -> ()  [unwired: 1 in, 6 out]
            n729 = local write "UserLevel"(0) -> ()
            n730 = local write "UserLogged"("") -> ()
            n731 = property on="PLC Connection Array" class="Arr (strict)"("DisabledEnum"=w952) -> ()  [unwired: 2 in, 2 out]
            n732 = property on="ResetAlarmButton" class="Bool"("Visible"=FALSE) -> ()  [unwired: 2 in, 2 out]
            n733 = property on="CountersConfigArray" class="Arr (strict)"("DisabledEnum"=w952) -> ()  [unwired: 2 in, 2 out]
            n734 = local read "GeneralParametersArray"() -> (w944:cluster{"Parameter":string, "Value":string}[])
            n735 = local read "GeneralParametersArray"() -> (w943:cluster{"Parameter":string, "Value":string}[])
            n736 = local read "GeneralParametersArray"() -> (w949:cluster{"Parameter":string, "Value":string}[])
            n737 = call "ScanParameters.vi"("MainConfigurationArray"=w944, "Parameter"="LineName") -> ("Value"=w945:string)  [unwired: 9 in]
            n738 = call "ScanParameters.vi"("MainConfigurationArray"=w943, "Parameter"="SubAssembly") -> ("Value"=w946:string)  [unwired: 9 in]
            n739 = call "ScanParameters.vi"("MainConfigurationArray"=w949, "Parameter"="ConnectionDSN") -> ("Value"=w950:string)  [unwired: 9 in]
            n740 = Concatenate Strings("update \"", w945, "_userlogged\" set \"useroperations\"='0',\"userquality\"='0' where \"subassembly\"='", w946, "'") -> (w947:string)
            n741 = To Lower Case(string=w947) -> (all lower case string=w948:string)
            n742 = call "SQL_QueryNoReturn.vi"("SQL query"=w948, "ConnectionDSN"=w950) -> ()  [unwired: 10 in]
          }
          event "EditUser": Value Change {
            n743 = event-data() -> ()  [unwired: 1 in, 6 out]
            n744 = local read "GeneralParametersArray"() -> (w960:cluster{"Parameter":string, "Value":string}[])
            n745 = local read "GeneralParametersArray"() -> (w959:cluster{"Parameter":string, "Value":string}[])
            n746 = call "ScanParameters.vi"("MainConfigurationArray"=w960, "Parameter"="ConnectionDSN") -> ("Value"=w955:string)  [unwired: 9 in]
            n747 = call "ScanParameters.vi"("MainConfigurationArray"=w959, "Parameter"="UsersTable") -> ("Value"=w956:string)  [unwired: 9 in]
            n748 = call "SQL_EditUser.vi"("UsersTable"=w956, "ConnectionDSN"=w955) -> ()  [unwired: 8 in, 2 out]
          }
          event "stop": Value Change {
            n749 = event-data() -> ()  [unwired: 1 in, 6 out]
            n750 = Stop() -> ()  [unwired: 1 in]
          }
          event "MaintenanceLogin": Value Change {
            n751 = event-data() -> ()  [unwired: 1 in, 6 out]
            n752 = stacked-sequence {
              seq-local: [w961 _] -> [_ w1009]
              frame #0 {
                w965 = ","
                n753 = local read "GeneralParametersArray"() -> (w972:cluster{"Parameter":string, "Value":string}[])
                n754 = local read "GeneralParametersArray"() -> (w971:cluster{"Parameter":string, "Value":string}[])
                n755 = call "ScanParameters.vi"("MainConfigurationArray"=w972, "Parameter"="ConnectionDSN") -> ("Value"=w961:string)  [unwired: 9 in]
                n756 = call "ScanParameters.vi"("MainConfigurationArray"=w971, "Parameter"="UsersTable") -> ("Value"=w970:string)  [unwired: 9 in]
                n757 = call "SQL_Login_Maintenance.vi"("UsersTable"=w970, "ConnectionDSN"=w961) -> ("User"=w967:string)  [unwired: 8 in, 1 out]
                n758 = Match Pattern(string=w967, regular expression=w965) -> (after substring=w966:string)  [unwired: 1 in, 3 out]
                n759 = Match Pattern(string=w966, regular expression=w965) -> (before substring=w964:string)  [unwired: 1 in, 3 out]
                n760 = Equal?(x=w964, y="Maintenance") -> (x = y?=w962:bool)
                n761 = case shown="True" w962 {
                  tunnel: w961 -> [_ w984]
                  frame False {
                  }
                  frame True {
                    n762 = local read "GeneralParametersArray"() -> (w982:cluster{"Parameter":string, "Value":string}[])
                    n763 = local read "GeneralParametersArray"() -> (w981:cluster{"Parameter":string, "Value":string}[])
                    n764 = call "ScanParameters.vi"("MainConfigurationArray"=w982, "Parameter"="SubAssembly") -> ("Value"=w975:string)  [unwired: 9 in]
                    n765 = call "ScanParameters.vi"("MainConfigurationArray"=w981, "Parameter"="LineName") -> ("Value"=w978:string)  [unwired: 9 in]
                    n766 = Concatenate Strings("update \"", w978, "_userlogged\" set \"useroperations\"='1' where \"subassembly\"='", w975, "'") -> (w974:string)
                    n767 = To Lower Case(string=w974) -> (all lower case string=w973:string)
                    n768 = call "SQL_QueryNoReturn.vi"("SQL query"=w973, "ConnectionDSN"=w984) -> ()  [unwired: 10 in]
                  }
                }
              }
              frame #1 {
                w988 = "1"
                n769 = local read "GeneralParametersArray"() -> (w1008:cluster{"Parameter":string, "Value":string}[])
                n770 = local read "GeneralParametersArray"() -> (w1003:cluster{"Parameter":string, "Value":string}[])
                n771 = call "ScanParameters.vi"("MainConfigurationArray"=w1008, "Parameter"="LineName") -> ("Value"=w1005:string)  [unwired: 9 in]
                n772 = call "ScanParameters.vi"("MainConfigurationArray"=w1003, "Parameter"="SubAssembly") -> ("Value"=w1001:string)  [unwired: 9 in]
                n773 = Concatenate Strings("select * from \"" ("SQL query"), w1005, "_userlogged\" where \"subassembly\"='", w1001, "'") -> (w999:string)
                n774 = To Lower Case(string=w999) -> (all lower case string=w998:string)
                n775 = call "SQL_QueryReturn.vi"("SQL query"=w998, "ConnectionDSN"=w1009) -> ("data"=w992:string[][])  [unwired: 9 in]
                n776 = Index Array(array=w992, index (col)=2 ("disabled index (col)")) -> (element=w991:string[])  [unwired: 1 in]
                n777 = Index Array(array=w992, index (col)=1 ("disabled index (col)")) -> (element=w996:string[])  [unwired: 1 in]
                n778 = Index Array(array=w991, index=0 ("disabled index (col)")) -> (element=w989:string)
                n779 = Index Array(array=w996, index=0 ("disabled index (col)")) -> (element=w990:string)
                n780 = Equal?(x=w990, y=w988) -> (x = y?=w987:bool)
                n781 = Equal?(x=w988, y=w989) -> (x = y?=w986:bool)
                n782 = And(x=w987, y=w986) -> (x .and. y?=w985:bool)
                n783 = case shown="True" w985 {
                  tunnel: w985 -> [_ w1011]
                  frame False {
                  }
                  frame True {
                    n784 = property on="ResetAlarmButton" class="Bool"("Visible"=w1011) -> ()  [unwired: 2 in, 2 out]
                    n785 = local read "Hour"() -> (w1010:string)
                    n786 = local write "HourResetEnabled"(w1010) -> ()
                  }
                }
              }
            }
          }
          event "QualityLogin": Value Change {
            n787 = event-data() -> ()  [unwired: 1 in, 6 out]
            n788 = stacked-sequence {
              seq-local: [w1012 _] -> [_ w1037]
              frame #0 {
                w1015 = ","
                n789 = local read "GeneralParametersArray"() -> (w1023:cluster{"Parameter":string, "Value":string}[])
                n790 = local read "GeneralParametersArray"() -> (w1022:cluster{"Parameter":string, "Value":string}[])
                n791 = call "ScanParameters.vi"("MainConfigurationArray"=w1023, "Parameter"="ConnectionDSN") -> ("Value"=w1012:string)  [unwired: 9 in]
                n792 = call "ScanParameters.vi"("MainConfigurationArray"=w1022, "Parameter"="UsersTable") -> ("Value"=w1021:string)  [unwired: 9 in]
                n793 = call "SQL_Login.vi"("UsersTable"=w1021, "ConnectionDSN"=w1012) -> ("User"=w1020:string)  [unwired: 8 in, 1 out]
                n794 = Match Pattern(string=w1020, regular expression=w1015) -> (after substring=w1019:string)  [unwired: 1 in, 3 out]
                n795 = Match Pattern(string=w1019, regular expression=w1015) -> (before substring=w1018:string)  [unwired: 1 in, 3 out]
                n796 = Equal?(x=w1018, y="Quality") -> (x = y?=w1017:bool)
                n797 = case shown="True" w1017 {
                  tunnel: w1012 -> [_ w1035]
                  frame False {
                  }
                  frame True {
                    n798 = local read "GeneralParametersArray"() -> (w1033:cluster{"Parameter":string, "Value":string}[])
                    n799 = local read "GeneralParametersArray"() -> (w1032:cluster{"Parameter":string, "Value":string}[])
                    n800 = call "ScanParameters.vi"("MainConfigurationArray"=w1033, "Parameter"="SubAssembly") -> ("Value"=w1026:string)  [unwired: 9 in]
                    n801 = call "ScanParameters.vi"("MainConfigurationArray"=w1032, "Parameter"="LineName") -> ("Value"=w1029:string)  [unwired: 9 in]
                    n802 = Concatenate Strings("update \"", w1029, "_userlogged\" set \"userquality\"='1' where \"subassembly\"='", w1026, "'") -> (w1025:string)
                    n803 = To Lower Case(string=w1025) -> (all lower case string=w1024:string)
                    n804 = call "SQL_QueryNoReturn.vi"("SQL query"=w1024, "ConnectionDSN"=w1035) -> ()  [unwired: 10 in]
                  }
                }
              }
              frame #1 {
                w1047 = "1"
                n805 = local read "GeneralParametersArray"() -> (w1060:cluster{"Parameter":string, "Value":string}[])
                n806 = local read "GeneralParametersArray"() -> (w1058:cluster{"Parameter":string, "Value":string}[])
                n807 = call "ScanParameters.vi"("MainConfigurationArray"=w1060, "Parameter"="LineName") -> ("Value"=w1059:string)  [unwired: 9 in]
                n808 = call "ScanParameters.vi"("MainConfigurationArray"=w1058, "Parameter"="SubAssembly") -> ("Value"=w1057:string)  [unwired: 9 in]
                n809 = Concatenate Strings("select * from \"" ("SQL query"), w1059, "_userlogged\" where \"subassembly\"='", w1057, "'") -> (w1056:string)
                n810 = To Lower Case(string=w1056) -> (all lower case string=w1055:string)
                n811 = call "SQL_QueryReturn.vi"("SQL query"=w1055, "ConnectionDSN"=w1037) -> ("data"=w1053:string[][])  [unwired: 9 in]
                n812 = Index Array(array=w1053, index (col)=2 ("disabled index (col)")) -> (element=w1052:string[])  [unwired: 1 in]
                n813 = Index Array(array=w1053, index (col)=1 ("disabled index (col)")) -> (element=w1054:string[])  [unwired: 1 in]
                n814 = Index Array(array=w1052, index=0 ("disabled index (col)")) -> (element=w1050:string)
                n815 = Index Array(array=w1054, index=0 ("disabled index (col)")) -> (element=w1051:string)
                n816 = Equal?(x=w1051, y=w1047) -> (x = y?=w1049:bool)
                n817 = Equal?(x=w1047, y=w1050) -> (x = y?=w1048:bool)
                n818 = And(x=w1049, y=w1048) -> (x .and. y?=w1036:bool)
                n819 = case shown="True" w1036 {
                  selector: w1036 -> [_ w1061]
                  frame False {
                  }
                  frame True {
                    n820 = local read "Hour"() -> (w1062:string)
                    n821 = property on="ResetAlarmButton" class="Bool"("Visible"=w1061) -> ()  [unwired: 2 in, 2 out]
                    n822 = local write "HourResetEnabled"(w1062) -> ()
                  }
                }
              }
            }
          }
          event "SearchSpareParts": Value Change {
            n823 = event-data() -> ()  [unwired: 1 in, 6 out]
            n824 = call "SQL_SearchSpareParts.vi"() -> ("Description.Text"=w1064:string, "ToolCribPN.Text"=w1063:string)  [unwired: 9 in, 1 out]
            n825 = local write "Tool Crib PN"(w1063) -> ()
            n826 = local write "Description"(w1064) -> ()
          }
          event "Add Button": Value Change {
            n827 = event-data() -> ()  [unwired: 1 in, 6 out]
            n828 = local read "Tool Crib PN"() -> (w1069:string)
            n829 = local read "Description"() -> (w1068:string)
            n830 = local read "CountersConfigArray"() -> (w1072:T5)
            n831 = Array Size(array=w1072) -> (size(s)=w1065:i32)
            n832 = Index Array(array=w1072, index=0) -> (element=w1070:T21)
            n833 = Bundle By Name(cluster=w1070, "ToolCribPartNumber"=w1069, "ComponentName"=w1068) -> (w1067:T21)
            n834 = Insert Into Array(array=w1072, index=w1065, new element=w1067) -> (w1066:T5)
            n835 = local write "CountersConfigArray"(w1066) -> ()
          }
          event "CreateTables": Value Change {
            n836 = event-data() -> ()  [unwired: 1 in, 6 out]
            n837 = local read "GeneralParametersArray"() -> (w1077:cluster{"Parameter":string, "Value":string}[])
            n838 = local read "GeneralParametersArray"() -> (w1081:cluster{"Parameter":string, "Value":string}[])
            n839 = local read "GeneralParametersArray"() -> (w1075:cluster{"Parameter":string, "Value":string}[])
            n840 = call "ScanParameters.vi"("MainConfigurationArray"=w1077, "Parameter"="LineName") -> ("Value"=w1076:string)  [unwired: 9 in]
            n841 = call "ScanParameters.vi"("MainConfigurationArray"=w1081, "Parameter"="ConnectionDSN") -> ("Value"=w1079:string)  [unwired: 9 in]
            n842 = call "ScanParameters.vi"("MainConfigurationArray"=w1075, "Parameter"="SubAssembly") -> ("Value"=w1073:string)  [unwired: 9 in]
            n843 = call "SQL_CreateTables.vi"("SubAssembly"=w1073, "LineName"=w1076, "ConnectionDSN"=w1079) -> ()  [unwired: 9 in]
          }
        }
      }
      n844 = while {
        stop <- w296 stop-if-true
        # "This loop is in charge of monitor the \nconnection between system and machine"
        n845 = local read "PLC Connection Array"() -> (w294:T11)
        n846 = local read "GeneralParametersArray"() -> (w291:cluster{"Parameter":string, "Value":string}[])
        n847 = for {
          tunnel: w294 -> [w304] mode=indexing
          tunnel: [w301] -> w295 mode=indexing
          tunnel: [w297] -> w293 mode=indexing
          n848 = Unbundle By Name(w304) -> ("MachineName"=w298:string, "PLC Address"=w303:string)
          n849 = local read "CycleTimeCluster"() -> (w300:T6)
          n850 = local read "ConnectionCluster"() -> (w302:cluster{"Connection":bool, "MachineName":string})
          n851 = call "Ping.vi"("hostNameOrAddress"=w303) -> ("bolStatus"=w299:bool)  [unwired: 8 in, 2 out]
          n852 = Bundle By Name(cluster=w302, "MachineName"=w298, "Connection"=w299) -> (w301:cluster{"Connection":bool, "MachineName":string})
          n853 = Bundle By Name(cluster=w300, "MachineName"=w298, "Connection"=w299) -> (w297:T6)
        }
        n854 = call "ScanParameters.vi"("MainConfigurationArray"=w291, "Parameter"="NidecServer") -> ("Value"=w290:string)  [unwired: 9 in]
        n855 = call "Ping.vi"("hostNameOrAddress"=w290) -> ("bolStatus"=w289:bool)  [unwired: 8 in, 2 out]
        n856 = Select(t="Online", s=w289, f="Offline") -> (s? t:f=w288:string)
        n857 = local write "ServerConnectionStatus"(w288) -> ()
        n858 = local write "CycleTimeMonitor"(w293) -> ()
        n859 = local write "OnlineStations"(w295) -> ()
        n860 = local read "stop"() -> (w296:bool)
      }
      n861 = while {
        stop <- w251 stop-if-true
        # "This loop is in charge of couting cycles."
        n862 = local read "Array_BooleanMemoryPLC"() -> (w248:T4)
        n863 = local read "PLC Connection Array"() -> (w249:T11)
        n864 = local read "OnlineStations"() -> (w250:T15)
        n865 = for {
          tunnel: w250 -> [w264] mode=indexing
          tunnel: w249 -> [w262] mode=indexing
          tunnel: w248 -> [w256] mode=indexing
          tunnel: [w253] -> w247 mode=indexing
          # "Count Cycle"
          n866 = Unbundle By Name(w262) -> ("PLC Address"=w260:string, "MemoryNumber1"=w261:string, "MachineName"=w259:string)  [unwired: 1 out]
          n867 = Unbundle By Name(w264) -> ("Connection"=w263:bool)
          n868 = local read "Hour"() -> (w252:string)
          n869 = Unbundle By Name(w256) -> ("PLC_Signal"=w255:bool, "MachineName"=w254:string)
          n870 = case shown="False" w263 {
            tunnel: w261 -> [_ w268]
            tunnel: w260 -> [_ w269]
            tunnel: w259 -> [_ w273]
            tunnel: [w266 w275] -> w258
            tunnel: [w265 w273] -> w257
            tunnel: w255 -> [w266 w276]
            tunnel: w254 -> [w265 w274]
            tunnel: w252 -> [_ w267]
            frame False {
            }
            frame True {
              n871 = call "ReadPLC_Keyence.vi"("MemoryNumber"=w268, "IP Address"=w269) -> ("BoolRead"=w275:bool)  [unwired: 9 in]
              n872 = Equal?(x=w273, y=w274) -> (x = y?=w272:bool)
              n873 = Not Equal?(x=w275, y=w276) -> (x != y?=w271:bool)
              n874 = And(x=w271, y=w272) -> (x .and. y?=w270:bool)
              n875 = case shown="True" w270 {
                tunnel: w275 -> [_ w283]
                tunnel: w273 -> [_ w282]
                tunnel: w267 -> [_ w277]
                frame False {
                }
                frame True {
                  n876 = local read "Counters Monitor Array"() -> (w285:T16)
                  n877 = local read "CycleTimeArray"() -> (w281:T1)
                  n878 = local read "CycleTimeMonitor"() -> (w279:T12)
                  n879 = call "AddCounterWithPLCSignal.vi"("CycleTimeMonitorIN"=w279, "CycleTimeArrayIN"=w281, "Hour"=w277, "Counters Monitor Array IN"=w285, "MachineName"=w282, "PLC_Bool_IN"=w283) -> ("CycleTimeMonitorOUT"=w278:T12, "Counters Monitor Array OUT"=w284:T16, "CycleTimeArrayOUT"=w280:T1)  [unwired: 3 in]
                  n880 = local write "Counters Monitor Array"(w284) -> ()
                  n881 = local write "CycleTimeMonitor"(w278) -> ()
                  n882 = local write "CycleTimeArray"(w280) -> ()
                }
              }
            }
          }
          n883 = Bundle By Name(cluster=w256, "PLC_Signal"=w258, "MachineName"=w257) -> (w253:cluster{"PLC_Signal":bool, "MachineName":string})
        }
        n884 = local write "Array_BooleanMemoryPLC"(w247) -> ()
        n885 = local read "stop"() -> (w251:bool)
      }
    }
  }
